vi "accuire.vi"() -> ()   [LabVIEW 2011]
uses:
  GUI_Template/GUI_master/tcp_new_data_event.ctl
  GUI_Template/GUI_master/tcp new data cluster.ctl
  Ctrs/beam detection.ctl
  GUI_Beampointing_single_TRA/Ctrs/move.ctl
  <userlib>/_OpenG.lib/array/array.llb/Filter 1D Array with Scalar (String)__ogtk.vi
  <vilib>/Analysis/NI_AALBase.lvlib
panel:
  in  "Offset X stats":dbl[][](array[numeric])
  in  "Offset Y stats":dbl[][](array[numeric])
  out "move properties 3":T1[](array[typedef])
  out "move properties 2":T1[](array[typedef])
  out "Box":T2(array[cluster])
  in  "Tab Control 2":enum32{"Config ", "Main", "History"}(tab)=enum."Main"
  in  "motor config":T3 {"Motor CCD 12" items=["PA2_Input1", "PA2_Input2", "L2_TelInpFar", "L1_TelInpNear", "L4_TREXPASS1", "L5_TREXPass2", "L6_TREXPass3", "L7_TREXPass4", "L8_M10Leak", "B1_TelInput", "B2_TelLens1", "", "", "", "MBeamSplitterL", "Mdiode"]; "Motor CCD 11" items=["PA2_Input1", "PA2_Input2", "L2_TelInpFar", "L1_TelInpNear", "L4_TREXPASS1", "L5_TREXPass2", "L6_TREXPass3", "L7_TREXPass4", "L8_M10Leak", "B1_TelInput", "B2_TelLens1", "", "", "", "MBeamSplitterL", "Mdiode"]; "Motor CCD 10" items=["PA2_Input1", "PA2_Input2", "L2_TelInpFar", "L1_TelInpNear", "L4_TREXPASS1", "L5_TREXPass2", "L6_TREXPass3", "L7_TREXPass4", "L8_M10Leak", "B1_TelInput", "B2_TelLens1", "", "", "", "MBeamSplitterL", "Mdiode"]; "Motor CCD 9" items=["PA2_Input1", "PA2_Input2", "L2_TelInpFar", "L1_TelInpNear", "L4_TREXPASS1", "L5_TREXPass2", "L6_TREXPass3", "L7_TREXPass4", "L8_M10Leak", "B1_TelInput", "B2_TelLens1", "", "", "", "MBeamSplitterL", "Mdiode"]; "Motor CCD 8" items=["PA2_Input1", "PA2_Input2", "L2_TelInpFar", "L1_TelInpNear", "L4_TREXPASS1", "L5_TREXPass2", "L6_TREXPass3", "L7_TREXPass4", "L8_M10Leak", "B1_TelInput", "B2_TelLens1", "", "", "", "MBeamSplitterL", "Mdiode"]; "Motor CCD 7" items=["PA2_Input1", "PA2_Input2", "L2_TelInpFar", "L1_TelInpNear", "L4_TREXPASS1", "L5_TREXPass2", "L6_TREXPass3", "L7_TREXPass4", "L8_M10Leak", "B1_TelInput", "B2_TelLens1", "", "", "", "MBeamSplitterL", "Mdiode"]; "Motor CCD 6" items=["PA2_Input1", "PA2_Input2", "L2_TelInpFar", "L1_TelInpNear", "L4_TREXPASS1", "L5_TREXPass2", "L6_TREXPass3", "L7_TREXPass4", "L8_M10Leak", "B1_TelInput", "B2_TelLens1", "", "", "", "MBeamSplitterL", "Mdiode"]; "Motor CCD 5" items=["PA2_Input1", "PA2_Input2", "L2_TelInpFar", "L1_TelInpNear", "L4_TREXPASS1", "L5_TREXPass2", "L6_TREXPass3", "L7_TREXPass4", "L8_M10Leak", "B1_TelInput", "B2_TelLens1", "", "", "", "MBeamSplitterL", "Mdiode"]; "Motor CCD 4" items=["PA2_Input1", "PA2_Input2", "L2_TelInpFar", "L1_TelInpNear", "L4_TREXPASS1", "L5_TREXPass2", "L6_TREXPass3", "L7_TREXPass4", "L8_M10Leak", "B1_TelInput", "B2_TelLens1", "", "", "", "MBeamSplitterL", "Mdiode"]; "Motor CCD 3" items=["PA2_Input1", "PA2_Input2", "L2_TelInpFar", "L1_TelInpNear", "L4_TREXPASS1", "L5_TREXPass2", "L6_TREXPass3", "L7_TREXPass4", "L8_M10Leak", "B1_TelInput", "B2_TelLens1", "", "", "", "MBeamSplitterL", "Mdiode"]; "Motor CCD 2" items=["PA2_Input1", "PA2_Input2", "L2_TelInpFar", "L1_TelInpNear", "L4_TREXPASS1", "L5_TREXPass2", "L6_TREXPass3", "L7_TREXPass4", "L8_M10Leak", "B1_TelInput", "B2_TelLens1", "", "", "", "MBeamSplitterL", "Mdiode"]; "Motor CCD 1" items=["PA2_Input1", "PA2_Input2", "L2_TelInpFar", "L1_TelInpNear", "L4_TREXPASS1", "L5_TREXPass2", "L6_TREXPass3", "L7_TREXPass4", "L8_M10Leak", "B1_TelInput", "B2_TelLens1", "", "", "", "MBeamSplitterL", "Mdiode"]}
  out "CCDs 2":T4
  out "sorted array X":cluster{dbl, "GUIdevice 7":string}[](array[cluster])
  out "sorted array Y":cluster{dbl, "GUIdevice 7":string}[](array[cluster])
  in  "Exposure::7":dbl=0.095 min=0.0001 max=1.0 format="%#_6f"
  in  "Triggerdelay::6":dbl=0.003 min=0.0 max=0.09 format="%#_6f"
  in  "Trigger::7":bool
  in  "Exposure::6":dbl=0.095 min=0.0001 max=1.0 format="%#_6f"
  in  "Triggerdelay::6":dbl=0.003 min=0.0 max=0.09 format="%#_6f"
  in  "Trigger::6":bool
  in  "Exposure::5":dbl=0.095 min=0.0001 max=1.0 format="%#_6f"
  in  "Triggerdelay::5":dbl=0.003 min=0.0 max=0.09 format="%#_6f"
  in  "Trigger::5":bool
  in  "Exposure::4":dbl=0.095 min=0.01 max=1.0 format="%#_6f"
  in  "Triggerdelay::4":dbl=0.003 min=0.0 max=0.09 format="%#_6f"
  in  "Trigger::4":bool
  in  "Exposure::3":dbl=0.095 min=0.0001 max=1.0 format="%#_6f"
  in  "Triggerdelay::3":dbl=0.003 min=0.0 max=0.09 format="%#_6f"
  in  "Trigger::3":bool
  in  "Exposure::2":dbl=0.095 min=0.0001 max=1.0 format="%#_6f"
  in  "Triggerdelay::2":dbl=0.003 min=0.0 max=0.09 format="%#_6f"
  in  "Trigger::2":bool
  out "image::1":T5(plugin-control) caption="L4_TREXpass1"
  out "image::2":T5(plugin-control) caption="L5_TREXPass2"
  out "image::3":T5(plugin-control) caption="L6_TREXpass3"
  out "image::4":T5(plugin-control) caption="L7_TREXPass4"
  out "image::5":T5(plugin-control) caption="L8_M10Leak"
  out "image::6":T5(plugin-control) caption="B1_TelInput"
  out "image::7":T5(plugin-control) caption="B2_TelLens1"
  out "Waveform Graph":cluster{i32, i32, "Centroid X":dbl[][]}(graph)
  out "image::8":T5(plugin-control)
  in  "Exposure::1":dbl=0.095 min=0.0001 max=1.0 format="%#_6f"
  in  "Triggerdelay::1":dbl=0.003 min=0.0 max=0.09 format="%#_6f"
  in  "Trigger::1":bool
  in  "UDP error message":string
  out "required Y":bool[](array[boolean])
  out "required X":bool[](array[boolean])
  out "detected":bool[](array[boolean])
  out "array":string[](array[string])
  out "CCD 5":cluster{timestamp[], dbl[]}[](graph)
  out "CCD 6":cluster{timestamp[], dbl[]}[](graph)
  out "CCD 7":cluster{timestamp[], dbl[]}[](graph)
  out "CCD 8":cluster{timestamp[], dbl[]}[](graph)
  out "CCD 1":cluster{timestamp[], dbl[]}[](graph)
  out "CCD 2":cluster{timestamp[], dbl[]}[](graph)
  out "CCD 3":cluster{timestamp[], dbl[]}[](graph)
  out "CCD 4":cluster{timestamp[], dbl[]}[](graph)
  in  "output cluster 2":T8 {"detection para"."smal para"."Measurement Parameter" items=["Center of Mass X", "Center of Mass Y", "First Pixel X", "First Pixel Y", "Bounding Rect Left", "Bounding Rect Top", "Bounding Rect Right", "Bounding Rect Bottom", "Max Feret Diameter Start X", "Max Feret Diameter Start Y", "Max Feret Diameter End X", "Max Feret Diameter End Y", "Max Horiz. Segment Length Left", "Max Horiz. Segment Length Right", "Max Horiz. Segment Length Row", "-", "Bounding Rect Width", "Bounding Rect Height", "Bounding Rect Diagonal", "Perimeter", "Convex Hull Perimeter", "Holes' Perimeter", "Max Feret Diameter", "Equivalent Ellipse Major Axis", "Equivalent Ellipse Minor Axis", "Equivalent Ellipse Minor Axis (Feret)", "Equivalent Rect Long Side", "Equivalent Rect Short Side", "Equivalent Rect Diagonal", "Equivalent Rect Short Side (Feret)", "Average Horiz. Segment Length", "Average Vert. Segment Length", "Hydraulic Radius", "Waddel Disk Diameter", "-", "Area", "Holes' Area", "Particle & Holes' Area", "Convex Hull Area", "Image Area", "-", "Number of Holes", "Number of Horiz. Segments", "Number of Vert. Segments", "-", "Orientation", "Max Feret Diameter Orientation", "-", "% Area/Image Area", "% Area/(Particle & Holes' Area)", "Ratio of Equivalent Ellipse Axes", "Ratio of Equivalent Rect Sides", "-", "Elongation Factor", "Compactness Factor", "Heywood Circularity Factor", "Type Factor", "-", "Sum X", "Sum Y", "Sum XX", "Sum XY", "Sum YY", "Sum XXX", "Sum XXY", "Sum XYY", "Sum YYY", "-", "Moment of Inertia XX", "Moment of Inertia XY", "Moment of Inertia YY", "Moment of Inertia XXX", "Moment of Inertia XXY", "Moment of Inertia XYY", "Moment of Inertia YYY", "Norm. Moment of Inertia XX", "Norm. Moment of Inertia XY", "Norm. Moment of Inertia YY", "Norm. Moment of Inertia XXX", "Norm. Moment of Inertia XXY", "Norm. Moment of Inertia XYY", "Norm. Moment of Inertia YYY", "Hu Moment 1", "Hu Moment 2", "Hu Moment 3", "Hu Moment 4", "Hu Moment 5", "Hu Moment 6", "Hu Moment 7"]; "detection para"."smal para"."Range Lower Value" format="%.2f"; "detection para"."smal para"."Range Upper Value" format="%.2f"; "detection para"."detection method" items=["clustering", "entropy", "metric", "moments", "inter-class variance"]; "detection para"."Filter" items=["No Filter", "Median Filter", "Low Pass Filter"]}
  out "Array":errorcluster[](array[cluster])
  out "Particle Reports (Pixels)":T9(array[cluster])
  in  "Feedback Global":bool
  in  "detection para":T6[](array[typedef])=[{"Filter"=1, "Filter Para"={"X Size"=5, "Y Size"=5, "% Tolerance"=1}, "detection method"=4, "smal para"=[{"Measurement Parameter"=35, "Range Lower Value"=0.0, "Range Upper Value"=0.0, "Range"=TRUE, "Measurement Type"=FALSE}], "Remove small Objects"=TRUE, "Restrict to round Objects"=FALSE}, {"Filter"=1, "Filter Para"={"X Size"=5, "Y Size"=5, "% Tolerance"=1}, "detection method"=4, "smal para"=[{"Measurement Parameter"=35, "Range Lower Value"=0.0, "Range Upper Value"=500.0, "Range"=FALSE, "Measurement Type"=FALSE}], "Remove small Objects"=TRUE, "Restrict to round Objects"=FALSE}, {"Filter"=1, "Filter Para"={"X Size"=5, "Y Size"=5, "% Tolerance"=1}, "detection method"=4, "smal para"=[{"Measurement Parameter"=35, "Range Lower Value"=0.0, "Range Upper Value"=500.0, "Range"=TRUE, "Measurement Type"=FALSE}], "Remove small Objects"=TRUE, "Restrict to round Objects"=FALSE}, {"Filter"=1, "Filter Para"={"X Size"=5, "Y Size"=5, "% Tolerance"=1}, "detection method"=4, "smal para"=[{"Measurement Parameter"=35, "Range Lower Value"=0.0, "Range Upper Value"=500.0, "Range"=TRUE, "Measurement Type"=FALSE}], "Remove small Objects"=TRUE, "Restrict to round Objects"=FALSE}, {"Filter"=1, "Filter Para"={"X Size"=5, "Y Size"=5, "% Tolerance"=1}, "detection method"=4, "smal para"=[{"Measurement Parameter"=35, "Range Lower Value"=0.0, "Range Upper Value"=500.0, "Range"=TRUE, "Measurement Type"=FALSE}], "Remove small Objects"=TRUE, "Restrict to round Objects"=FALSE}, {"Filter"=1, "Filter Para"={"X Size"=5, "Y Size"=5, "% Tolerance"=1}, "detection method"=4, "smal para"=[{"Measurement Parameter"=35, "Range Lower Value"=0.0, "Range Upper Value"=500.0, "Range"=TRUE, "Measurement Type"=FALSE}], "Remove small Objects"=TRUE, "Restrict to round Objects"=FALSE}, {"Filter"=1, "Filter Para"={"X Size"=5, "Y Size"=5, "% Tolerance"=1}, "detection method"=4, "smal para"=[{"Measurement Parameter"=35, "Range Lower Value"=0.0, "Range Upper Value"=500.0, "Range"=TRUE, "Measurement Type"=FALSE}], "Remove small Objects"=TRUE, "Restrict to round Objects"=FALSE}, {"Filter"=1, "Filter Para"={"X Size"=5, "Y Size"=5, "% Tolerance"=1}, "detection method"=3, "smal para"=[{"Measurement Parameter"=35, "Range Lower Value"=0.0, "Range Upper Value"=0.0, "Range"=FALSE, "Measurement Type"=FALSE}], "Remove small Objects"=TRUE, "Restrict to round Objects"=FALSE}, {"Filter"=1, "Filter Para"={"X Size"=5, "Y Size"=5, "% Tolerance"=1}, "detection method"=4, "smal para"=[{"Measurement Parameter"=35, "Range Lower Value"=0.0, "Range Upper Value"=0.0, "Range"=FALSE, "Measurement Type"=FALSE}], "Remove small Objects"=TRUE, "Restrict to round Objects"=FALSE}, {"Filter"=1, "Filter Para"={"X Size"=5, "Y Size"=5, "% Tolerance"=1}, "detection method"=4, "smal para"=[{"Measurement Parameter"=35, "Range Lower Value"=0.0, "Range Upper Value"=500.0, "Range"=TRUE, "Measurement Type"=FALSE}], "Remove small Objects"=TRUE, "Restrict to round Objects"=FALSE}, {"Filter"=1, "Filter Para"={"X Size"=5, "Y Size"=5, "% Tolerance"=1}, "detection method"=4, "smal para"=[{"Measurement Parameter"=35, "Range Lower Value"=0.0, "Range Upper Value"=500.0, "Range"=TRUE, "Measurement Type"=FALSE}], "Remove small Objects"=TRUE, "Restrict to round Objects"=FALSE}, {"Filter"=1, "Filter Para"={"X Size"=5, "Y Size"=5, "% Tolerance"=1}, "detection method"=4, "smal para"=[{"Measurement Parameter"=35, "Range Lower Value"=0.0, "Range Upper Value"=500.0, "Range"=TRUE, "Measurement Type"=FALSE}], "Remove small Objects"=TRUE, "Restrict to round Objects"=FALSE}] {"smal para"."Measurement Parameter" items=["Center of Mass X", "Center of Mass Y", "First Pixel X", "First Pixel Y", "Bounding Rect Left", "Bounding Rect Top", "Bounding Rect Right", "Bounding Rect Bottom", "Max Feret Diameter Start X", "Max Feret Diameter Start Y", "Max Feret Diameter End X", "Max Feret Diameter End Y", "Max Horiz. Segment Length Left", "Max Horiz. Segment Length Right", "Max Horiz. Segment Length Row", "-", "Bounding Rect Width", "Bounding Rect Height", "Bounding Rect Diagonal", "Perimeter", "Convex Hull Perimeter", "Holes' Perimeter", "Max Feret Diameter", "Equivalent Ellipse Major Axis", "Equivalent Ellipse Minor Axis", "Equivalent Ellipse Minor Axis (Feret)", "Equivalent Rect Long Side", "Equivalent Rect Short Side", "Equivalent Rect Diagonal", "Equivalent Rect Short Side (Feret)", "Average Horiz. Segment Length", "Average Vert. Segment Length", "Hydraulic Radius", "Waddel Disk Diameter", "-", "Area", "Holes' Area", "Particle & Holes' Area", "Convex Hull Area", "Image Area", "-", "Number of Holes", "Number of Horiz. Segments", "Number of Vert. Segments", "-", "Orientation", "Max Feret Diameter Orientation", "-", "% Area/Image Area", "% Area/(Particle & Holes' Area)", "Ratio of Equivalent Ellipse Axes", "Ratio of Equivalent Rect Sides", "-", "Elongation Factor", "Compactness Factor", "Heywood Circularity Factor", "Type Factor", "-", "Sum X", "Sum Y", "Sum XX", "Sum XY", "Sum YY", "Sum XXX", "Sum XXY", "Sum XYY", "Sum YYY", "-", "Moment of Inertia XX", "Moment of Inertia XY", "Moment of Inertia YY", "Moment of Inertia XXX", "Moment of Inertia XXY", "Moment of Inertia XYY", "Moment of Inertia YYY", "Norm. Moment of Inertia XX", "Norm. Moment of Inertia XY", "Norm. Moment of Inertia YY", "Norm. Moment of Inertia XXX", "Norm. Moment of Inertia XXY", "Norm. Moment of Inertia XYY", "Norm. Moment of Inertia YYY", "Hu Moment 1", "Hu Moment 2", "Hu Moment 3", "Hu Moment 4", "Hu Moment 5", "Hu Moment 6", "Hu Moment 7"]; "smal para"."Range Lower Value" format="%.2f"; "smal para"."Range Upper Value" format="%.2f"; "detection method" items=["clustering", "entropy", "metric", "moments", "inter-class variance"]; "Filter" items=["No Filter", "Median Filter", "Low Pass Filter"]}
  in  "Target.X::8":dbl=47.0 min=0.0 max=2000.0 format="%#_6f"
  in  "Target.Y::8":dbl=45.0 min=0.0 max=2000.0 format="%#_6f"
  in  "GUIdevice 8":string
  in  "Tab Control":T10(tab)=enum."Detection"
  in  "Save Stats":bool
  in  "Save Config":bool
  in  "Load Config":bool
  in  "updat speed [ms]":i32=200
  in  "img to avg":i32=20
  in  "Reset History":bool
  in  "beam detection para":T6={"Filter"=1, "Filter Para"={"X Size"=5, "Y Size"=5, "% Tolerance"=1}, "detection method"=4, "smal para"=[{"Measurement Parameter"=35, "Range Lower Value"=0.0, "Range Upper Value"=500.0, "Range"=FALSE, "Measurement Type"=FALSE}], "Remove small Objects"=TRUE, "Restrict to round Objects"=FALSE} {"smal para"."Measurement Parameter" items=["Center of Mass X", "Center of Mass Y", "First Pixel X", "First Pixel Y", "Bounding Rect Left", "Bounding Rect Top", "Bounding Rect Right", "Bounding Rect Bottom", "Max Feret Diameter Start X", "Max Feret Diameter Start Y", "Max Feret Diameter End X", "Max Feret Diameter End Y", "Max Horiz. Segment Length Left", "Max Horiz. Segment Length Right", "Max Horiz. Segment Length Row", "-", "Bounding Rect Width", "Bounding Rect Height", "Bounding Rect Diagonal", "Perimeter", "Convex Hull Perimeter", "Holes' Perimeter", "Max Feret Diameter", "Equivalent Ellipse Major Axis", "Equivalent Ellipse Minor Axis", "Equivalent Ellipse Minor Axis (Feret)", "Equivalent Rect Long Side", "Equivalent Rect Short Side", "Equivalent Rect Diagonal", "Equivalent Rect Short Side (Feret)", "Average Horiz. Segment Length", "Average Vert. Segment Length", "Hydraulic Radius", "Waddel Disk Diameter", "-", "Area", "Holes' Area", "Particle & Holes' Area", "Convex Hull Area", "Image Area", "-", "Number of Holes", "Number of Horiz. Segments", "Number of Vert. Segments", "-", "Orientation", "Max Feret Diameter Orientation", "-", "% Area/Image Area", "% Area/(Particle & Holes' Area)", "Ratio of Equivalent Ellipse Axes", "Ratio of Equivalent Rect Sides", "-", "Elongation Factor", "Compactness Factor", "Heywood Circularity Factor", "Type Factor", "-", "Sum X", "Sum Y", "Sum XX", "Sum XY", "Sum YY", "Sum XXX", "Sum XXY", "Sum XYY", "Sum YYY", "-", "Moment of Inertia XX", "Moment of Inertia XY", "Moment of Inertia YY", "Moment of Inertia XXX", "Moment of Inertia XXY", "Moment of Inertia XYY", "Moment of Inertia YYY", "Norm. Moment of Inertia XX", "Norm. Moment of Inertia XY", "Norm. Moment of Inertia YY", "Norm. Moment of Inertia XXX", "Norm. Moment of Inertia XXY", "Norm. Moment of Inertia XYY", "Norm. Moment of Inertia YYY", "Hu Moment 1", "Hu Moment 2", "Hu Moment 3", "Hu Moment 4", "Hu Moment 5", "Hu Moment 6", "Hu Moment 7"]; "smal para"."Range Lower Value" format="%.2f"; "smal para"."Range Upper Value" format="%.2f"; "detection method" items=["clustering", "entropy", "metric", "moments", "inter-class variance"]; "Filter" items=["No Filter", "Median Filter", "Low Pass Filter"]}
  in  "move config":T1={"Tolerance [%]"=0.1, "Stepsize"=0.0001, "Invert Axis"=TRUE, "Invert Direction X"=FALSE, "Invert Direction Y"=TRUE, "enable feedback"=FALSE, "my activ motor"=""}
  out "Arguments Y":string
  in  "active axis refs 2":T11(array[cluster])
  in  "active Axis ref":cluster{"Ref X":refnum<vi>, "Ref Y":refnum<vi>}
  in  "CCDs":u16(ring) items=["L4_TREXpass1", "L5_TREXPass2", "L6_TREXpass3", "L7_TREXPass4", "L8_M10Leak", "B1_TelInput", "B2_TelLens1", ""]
  out "motor refs":refnum<vi>[](array[refnum])
  in  "Position.Axis 511::99":dbl=77.0 caption="Motor Axis 1" min=-999999.0 max=999999.0 format="%#_6f"
  in  "Position.Axis 512::99":dbl=77.0 caption="Motor Axis 1" min=-999999.0 max=999999.0 format="%#_6f"
  in  "Position.Axis 513::99":dbl=77.0 caption="Motor Axis 1" min=-999999.0 max=999999.0 format="%#_6f"
  in  "Position.Axis 521::99":dbl=77.0 caption="Motor Axis 1" min=-999999.0 max=999999.0 format="%#_6f"
  in  "Position.Axis 522::99":dbl=77.0 caption="Motor Axis 1" min=-999999.0 max=999999.0 format="%#_6f"
  in  "Position.Axis 523::99":dbl=77.0 caption="Motor Axis 1" min=-999999.0 max=999999.0 format="%#_6f"
  in  "Position.Axis 531::99":dbl=77.0 caption="Motor Axis 1" min=-999999.0 max=999999.0 format="%#_6f"
  in  "Position.Axis 532::99":dbl=77.0 caption="Motor Axis 1" min=-999999.0 max=999999.0 format="%#_6f"
  in  "Position.Axis 533::99":dbl=77.0 caption="Motor Axis 1" min=-999999.0 max=999999.0 format="%#_6f"
  in  "Position.Axis 541::99":dbl=77.0 caption="Motor Axis 1" min=-999999.0 max=999999.0 format="%#_6f"
  in  "Position.Axis 542::99":dbl=77.0 caption="Motor Axis 1" min=-999999.0 max=999999.0 format="%#_6f"
  in  "Position.Axis 543::99":dbl=77.0 caption="Motor Axis 1" min=-999999.0 max=999999.0 format="%#_6f"
  in  "Position.Axis 411::99":dbl=77.0 caption="Motor Axis 1" min=-999999.0 max=999999.0 format="%#_6f"
  in  "Position.Axis 412::99":dbl=77.0 caption="Motor Axis 1" min=-999999.0 max=999999.0 format="%#_6f"
  in  "Position.Axis 413::99":dbl=77.0 caption="Motor Axis 1" min=-999999.0 max=999999.0 format="%#_6f"
  in  "Position.Axis 421::99":dbl=77.0 caption="Motor Axis 1" min=-999999.0 max=999999.0 format="%#_6f"
  in  "Position.Axis 422::99":dbl=77.0 caption="Motor Axis 1" min=-999999.0 max=999999.0 format="%#_6f"
  in  "Position.Axis 423::99":dbl=77.0 caption="Motor Axis 1" min=-999999.0 max=999999.0 format="%#_6f"
  in  "Position.Axis 431::99":dbl=77.0 caption="Motor Axis 1" min=-999999.0 max=999999.0 format="%#_6f"
  in  "Position.Axis 432::99":dbl=77.0 caption="Motor Axis 1" min=-999999.0 max=999999.0 format="%#_6f"
  in  "Position.Axis 433::99":dbl=77.0 caption="Motor Axis 1" min=-999999.0 max=999999.0 format="%#_6f"
  in  "Position.Axis 441::99":dbl=77.0 caption="Motor Axis 1" min=-999999.0 max=999999.0 format="%#_6f"
  in  "Position.Axis 442::99":dbl=77.0 caption="Motor Axis 1" min=-999999.0 max=999999.0 format="%#_6f"
  in  "Position.Axis 443::99":dbl=77.0 caption="Motor Axis 1" min=-999999.0 max=999999.0 format="%#_6f"
  in  "Position.Axis 311::99":dbl=77.0 caption="Motor Axis 1" min=-999999.0 max=999999.0 format="%#_6f"
  in  "Position.Axis 312::99":dbl=77.0 caption="Motor Axis 1" min=-999999.0 max=999999.0 format="%#_6f"
  in  "Position.Axis 313::99":dbl=77.0 caption="Motor Axis 1" min=-999999.0 max=999999.0 format="%#_6f"
  in  "Position.Axis 321::99":dbl=77.0 caption="Motor Axis 1" min=-999999.0 max=999999.0 format="%#_6f"
  in  "Position.Axis 322::99":dbl=77.0 caption="Motor Axis 1" min=-999999.0 max=999999.0 format="%#_6f"
  in  "Position.Axis 323::99":dbl=77.0 caption="Motor Axis 1" min=-999999.0 max=999999.0 format="%#_6f"
  in  "Position.Axis 331::99":dbl=77.0 caption="Motor Axis 1" min=-999999.0 max=999999.0 format="%#_6f"
  in  "Position.Axis 332::99":dbl=77.0 caption="Motor Axis 1" min=-999999.0 max=999999.0 format="%#_6f"
  in  "Position.Axis 333::99":dbl=77.0 caption="Motor Axis 1" min=-999999.0 max=999999.0 format="%#_6f"
  in  "Position.Axis 341::99":dbl=77.0 caption="Motor Axis 1" min=-999999.0 max=999999.0 format="%#_6f"
  in  "Position.Axis 342::99":dbl=77.0 caption="Motor Axis 1" min=-999999.0 max=999999.0 format="%#_6f"
  in  "Position.Axis 343::99":dbl=77.0 caption="Motor Axis 1" min=-999999.0 max=999999.0 format="%#_6f"
  in  "Position.Axis 241::99":dbl=77.0 caption="Motor Axis 1" min=-999999.0 max=999999.0 format="%#_6f"
  in  "Position.Axis 242::99":dbl=77.0 caption="Motor Axis 1" min=-999999.0 max=999999.0 format="%#_6f"
  in  "Position.Axis 243::99":dbl=77.0 caption="Motor Axis 1" min=-999999.0 max=999999.0 format="%#_6f"
  in  "Position.Axis 231::99":dbl=77.0 caption="Motor Axis 1" min=-999999.0 max=999999.0 format="%#_6f"
  in  "Position.Axis 232::99":dbl=77.0 caption="Motor Axis 1" min=-999999.0 max=999999.0 format="%#_6f"
  in  "Position.Axis 233::99":dbl=77.0 caption="Motor Axis 1" min=-999999.0 max=999999.0 format="%#_6f"
  in  "Position.Axis 221::99":dbl=77.0 caption="Motor Axis 1" min=-20000.0 max=20000.0 format="%#_6f"
  in  "Position.Axis 222::99":dbl=77.0 caption="Motor Axis 1" min=-200000.0 max=200000.0 format="%#_6f"
  in  "Position.Axis 223::99":dbl=77.0 caption="Motor Axis 1" min=-20000.0 max=200000000.0 format="%#_6f"
  in  "Position.Axis 211::99":dbl=77.0 caption="Motor Axis 1" min=-200000.0 max=2000000.0 format="%#_6f"
  in  "Position.Axis 212::99":dbl=77.0 caption="Motor Axis 1" min=-200000.0 max=2000.0 format="%#_6f"
  in  "Position.Axis 213::99":dbl=77.0 caption="Motor Axis 1" min=-2000.0 max=2000000.0 format="%#_6f"
  in  "Position.Axis 141::99":dbl=77.0 caption="Motor Axis 1" min=-999999.0 max=999999.0 format="%#_6f"
  in  "Position.Axis 142::99":dbl=77.0 caption="Motor Axis 1" min=-999999.0 max=999999.0 format="%#_6f"
  in  "Position.Axis 143::99":dbl=77.0 caption="Motor Axis 1" min=-999999.0 max=999999.0 format="%#_6f"
  in  "Position.Axis 131::99":dbl=77.0 caption="Motor Axis 1" min=-999999.0 max=999999.0 format="%#_6f"
  in  "Position.Axis 132::99":dbl=77.0 caption="Motor Axis 1" min=-999999.0 max=999999.0 format="%#_6f"
  in  "Position.Axis 133::99":dbl=77.0 caption="Motor Axis 1" min=-999999.0 max=999999.0 format="%#_6f"
  in  "Position.Axis 121::99":dbl=77.0 caption="Motor Axis 1" min=-999999.0 max=999999.0 format="%#_6f"
  in  "Position.Axis 122::99":dbl=77.0 caption="Motor Axis 1" min=-999999.0 max=999999.0 format="%#_6f"
  in  "Position.Axis 123::99":dbl=77.0 caption="Motor Axis 1" min=-999999.0 max=999999.0 format="%#_6f"
  in  "Position.Axis 113::99":dbl=77.0 caption="Motor Axis 1" min=-999999.0 max=999999.0 format="%#_6f"
  in  "Position.Axis 112::99":dbl=77.0 caption="Motor Axis 1" min=-999999.0 max=999999.0 format="%#_6f"
  in  "Position.Axis 111::99":dbl=77.0 caption="Motor Axis 1" min=-999999.0 max=999999.0 format="%#_6f"
  out "Arguments X":string
  in  "GUIdevice 99":string="PicoPad3"
  in  "move properties":T1[](array[typedef])=[{"Tolerance [%]"=5.0, "Stepsize"=5.0, "Invert Axis"=FALSE, "Invert Direction X"=FALSE, "Invert Direction Y"=FALSE, "enable feedback"=FALSE, "my activ motor"=""}, {"Tolerance [%]"=5.0, "Stepsize"=5.0, "Invert Axis"=FALSE, "Invert Direction X"=FALSE, "Invert Direction Y"=FALSE, "enable feedback"=FALSE, "my activ motor"=""}, {"Tolerance [%]"=5.0, "Stepsize"=5.0, "Invert Axis"=FALSE, "Invert Direction X"=FALSE, "Invert Direction Y"=FALSE, "enable feedback"=FALSE, "my activ motor"=""}, {"Tolerance [%]"=5.0, "Stepsize"=5.0, "Invert Axis"=FALSE, "Invert Direction X"=FALSE, "Invert Direction Y"=FALSE, "enable feedback"=FALSE, "my activ motor"=""}, {"Tolerance [%]"=5.0, "Stepsize"=5.0, "Invert Axis"=FALSE, "Invert Direction X"=FALSE, "Invert Direction Y"=FALSE, "enable feedback"=FALSE, "my activ motor"=""}, {"Tolerance [%]"=5.0, "Stepsize"=5.0, "Invert Axis"=FALSE, "Invert Direction X"=FALSE, "Invert Direction Y"=FALSE, "enable feedback"=FALSE, "my activ motor"=""}, {"Tolerance [%]"=5.0, "Stepsize"=5.0, "Invert Axis"=FALSE, "Invert Direction X"=FALSE, "Invert Direction Y"=FALSE, "enable feedback"=FALSE, "my activ motor"=""}, {"Tolerance [%]"=5.0, "Stepsize"=5.0, "Invert Axis"=FALSE, "Invert Direction X"=FALSE, "Invert Direction Y"=FALSE, "enable feedback"=FALSE, "my activ motor"=""}, {"Tolerance [%]"=5.0, "Stepsize"=5.0, "Invert Axis"=FALSE, "Invert Direction X"=FALSE, "Invert Direction Y"=FALSE, "enable feedback"=FALSE, "my activ motor"=""}, {"Tolerance [%]"=5.0, "Stepsize"=5.0, "Invert Axis"=FALSE, "Invert Direction X"=FALSE, "Invert Direction Y"=FALSE, "enable feedback"=FALSE, "my activ motor"=""}, {"Tolerance [%]"=5.0, "Stepsize"=5.0, "Invert Axis"=FALSE, "Invert Direction X"=FALSE, "Invert Direction Y"=FALSE, "enable feedback"=FALSE, "my activ motor"=""}, {"Tolerance [%]"=5.0, "Stepsize"=5.0, "Invert Axis"=FALSE, "Invert Direction X"=FALSE, "Invert Direction Y"=FALSE, "enable feedback"=FALSE, "my activ motor"=""}, {"Tolerance [%]"=5.0, "Stepsize"=5.0, "Invert Axis"=FALSE, "Invert Direction X"=FALSE, "Invert Direction Y"=FALSE, "enable feedback"=FALSE, "my activ motor"=""}]
  in  "Time":timestamp[][](array[timestamp])
  in  "Mean Size":dbl[][](array[numeric])
  in  "Size":dbl[][](array[numeric])
  in  "active CCDs":i32(listbox)=1
  in  "Offset Y":dbl[][](array[numeric])
  in  "Offset X":dbl[][](array[numeric])
  in  "Mean Centroid X":dbl[][](array[numeric])
  in  "Mean Centroid Y":dbl[][](array[numeric])
  in  "Centroid Y":dbl[][](array[numeric])
  in  "Centroid X":dbl[][](array[numeric])
  in  "Target.X::7":dbl=47.0 min=0.0 max=2000.0 format="%#_6f"
  in  "Target.Y::7":dbl=45.0 min=0.0 max=2000.0 format="%#_6f"
  in  "Target.X::6":dbl=47.0 min=0.0 max=2000.0 format="%#_6f"
  in  "Target.Y::6":dbl=45.0 min=0.0 max=2000.0 format="%#_6f"
  in  "Target.X::5":dbl=47.0 min=0.0 max=2000.0 format="%#_6f"
  in  "Target.Y::5":dbl=45.0 min=0.0 max=2000.0 format="%#_6f"
  in  "Target.X::4":dbl=47.0 min=0.0 max=2000.0 format="%#_6f"
  in  "Target.Y::4":dbl=45.0 min=0.0 max=2000.0 format="%#_6f"
  in  "Target.X::3":dbl=152.0 min=0.0 max=2000.0 format="%#_6f"
  in  "Target.Y::3":dbl=163.0 min=0.0 max=2000.0 format="%#_6f"
  in  "Target.X::2":dbl=75.0 min=0.0 max=2000.0 format="%#_6f"
  in  "Target.Y::2":dbl=74.0 min=0.0 max=2000.0 format="%#_6f"
  in  "Target.X::1":dbl=77.0 min=0.0 max=2000.0 format="%#_6f"
  in  "Target.Y::1":dbl=61.0 min=0.0 max=2000.0 format="%#_6f"
  in  "GUIdevice 7":string="B2_TelLens1"
  in  "GUIdevice 6":string="B1_TelInput"
  in  "GUIdevice 5":string="L8_M10Leak"
  in  "GUIdevice 4":string="L7_TREXPass4"
  in  "GUIdevice 3":string="L6_TREXpass3"
  in  "GUIdevice 2":string="L5_TREXPass2"
  in  "insert tag":bool=TRUE
  in  "stop":bool
  in  "GUIdevice 1":string="L4_TREXpass1"
  out "tcp data event":T12
  out "error IO 2":errorcluster
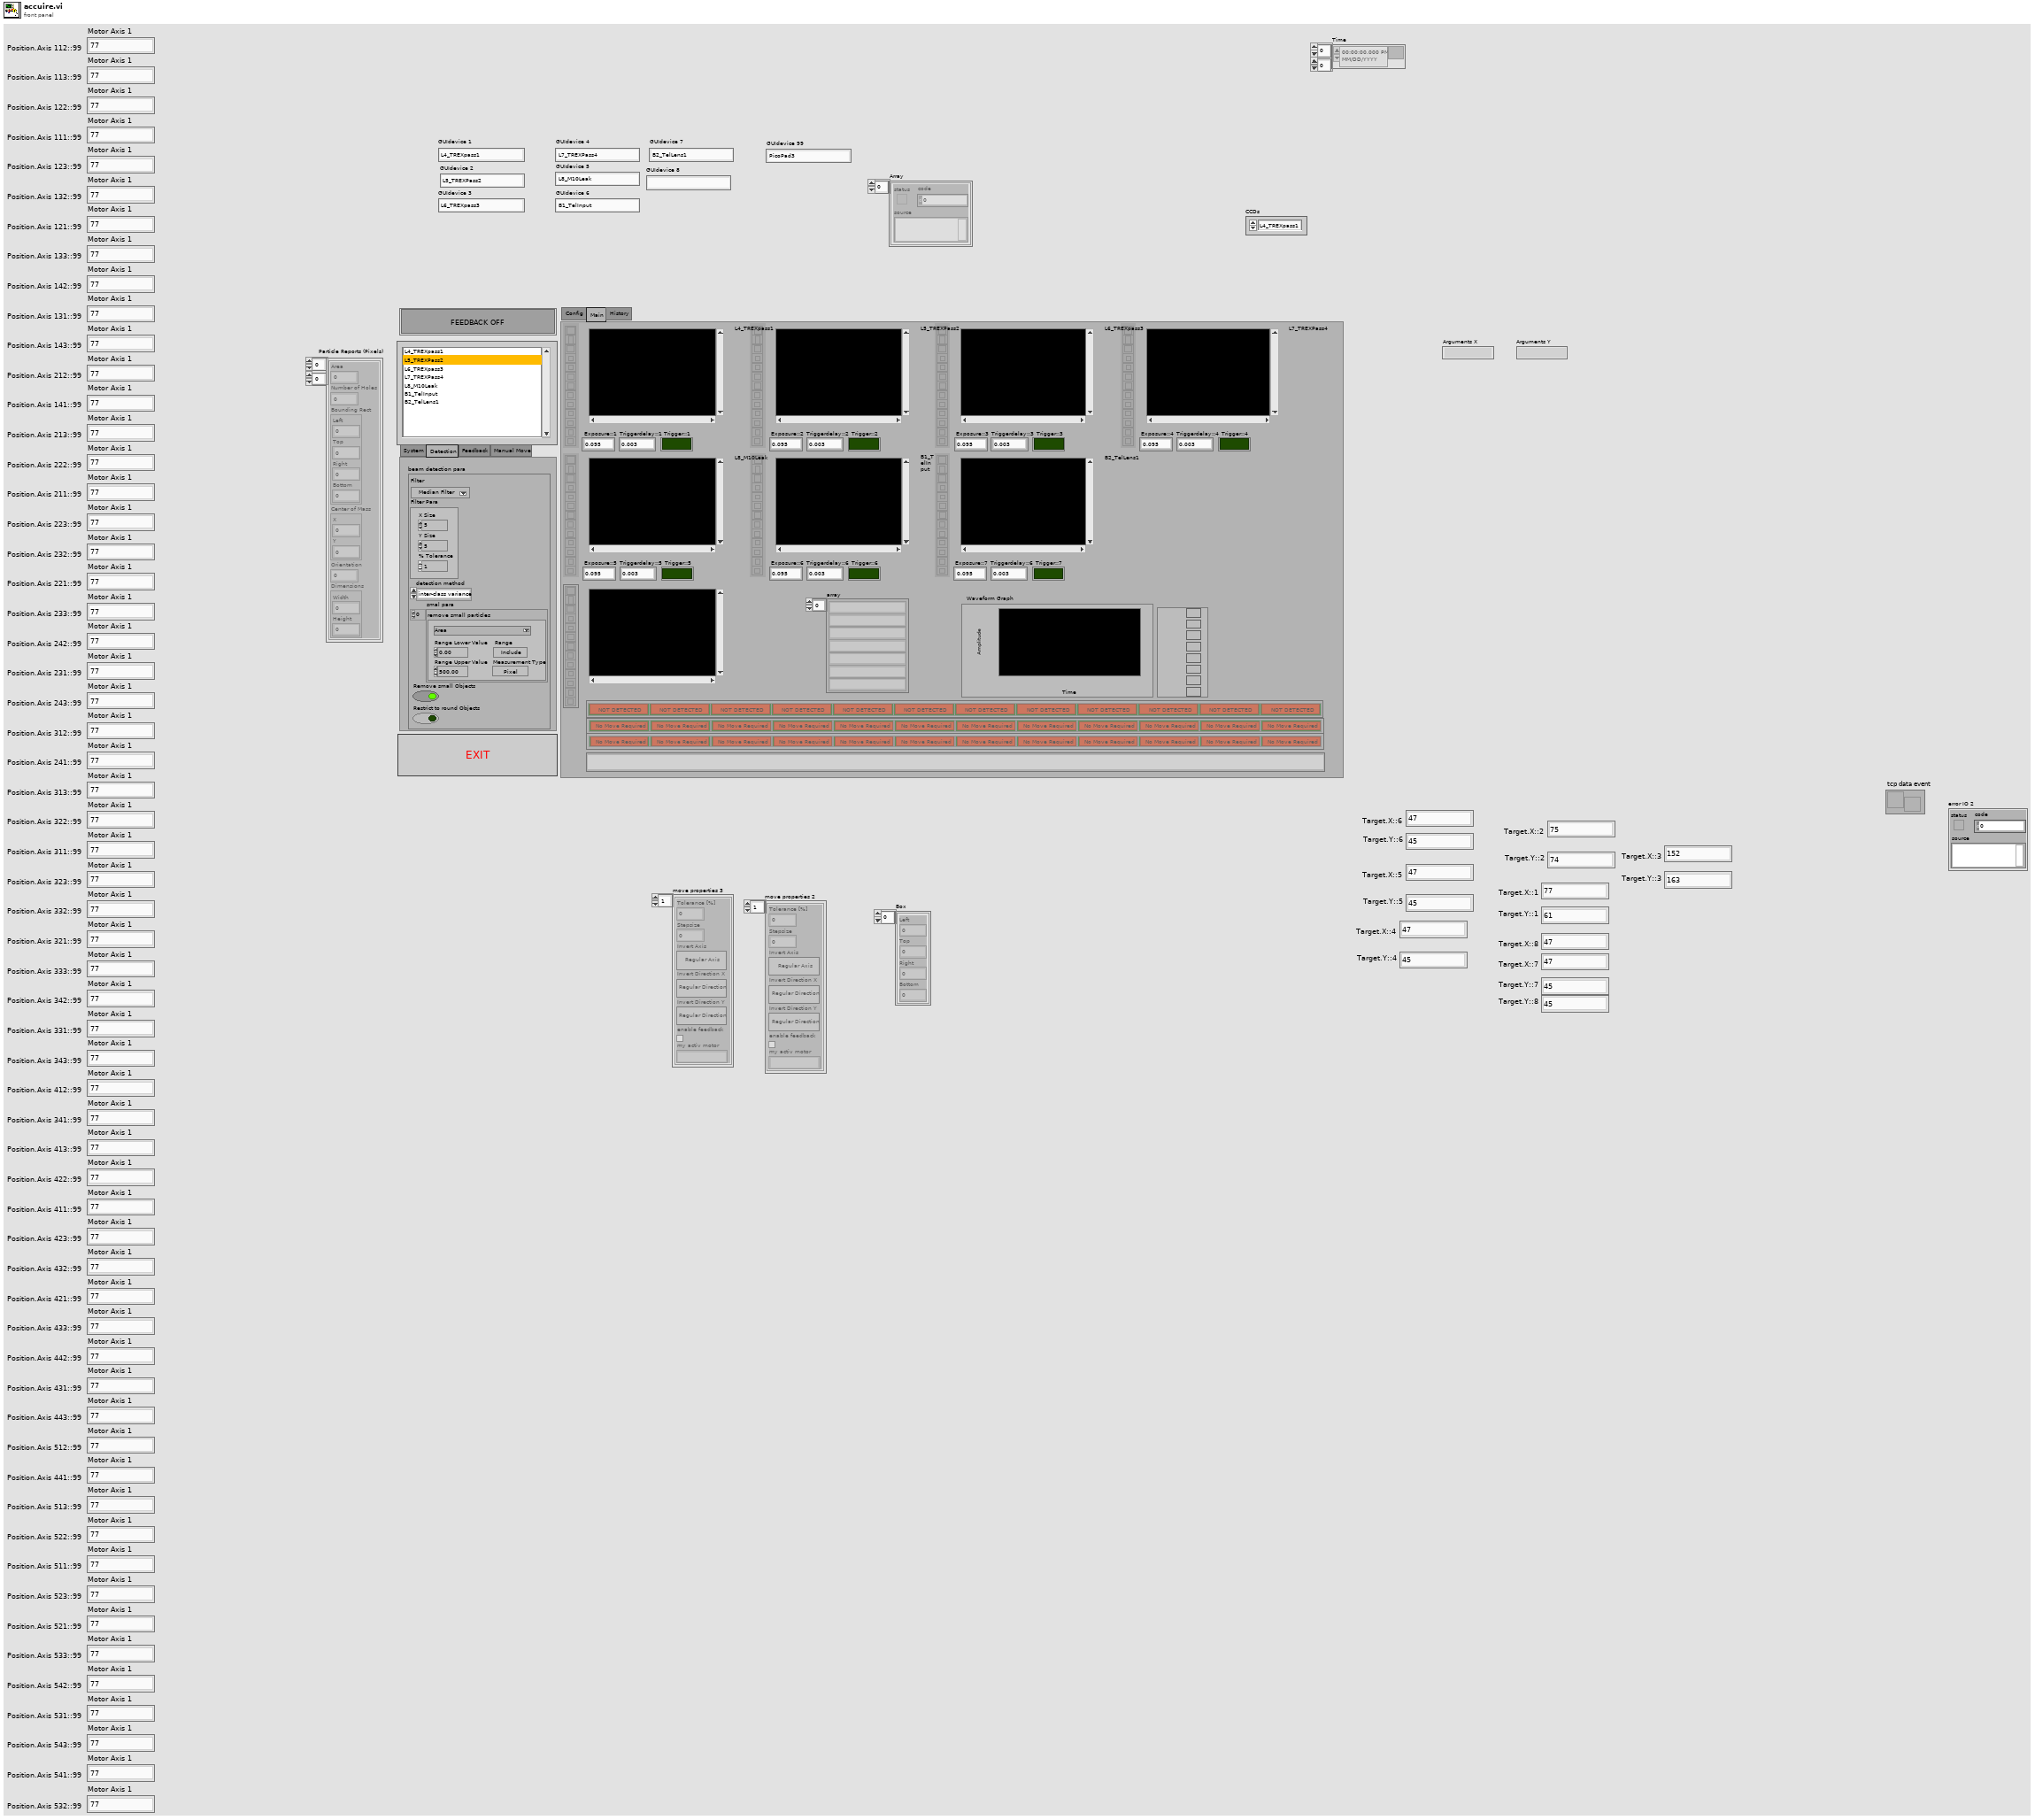
[diagram p1: front panel]
types:
  T1 = typedef "move.ctl" = cluster{"Tolerance [%]":dbl, "Stepsize":dbl, "Invert Axis":bool, "Invert Direction X":bool, "Invert Direction Y":bool, "enable feedback":bool, "my activ motor":string}
  T2 = cluster{"Left":dbl, "Top":dbl, "Right":dbl, "Bottom":dbl}[]
  T3 = cluster{"Motor CCD 1":u16, "Motor CCD 2":u16, "Motor CCD 3":u16, "Motor CCD 4":u16, "Motor CCD 5":u16, "Motor CCD 6":u16, "Motor CCD 7":u16, "Motor CCD 8":u16, "Motor CCD 9":u16, "Motor CCD 10":u16, "Motor CCD 11":u16, "Motor CCD 12":u16}
  T4 = cluster{"[0]":string, "[1]":string, "[2]":string, "[3]":string, "[4]":string, "[5]":string, "[6]":string, "[7]":string, "[8]":string}
  T5 = typedef "IMAQ Image.ctl" = refnum<image>
  T6 = typedef "beam detection.ctl" = cluster{"Filter":u16, "Filter Para":cluster{"X Size":i32, "Y Size":i32, "% Tolerance":i32}, "detection method":i32, "smal para":cluster{"Measurement Parameter":T7, "Range Lower Value":dbl, "Range Upper Value":dbl, "Range":bool, "Measurement Type":bool}[], "Remove small Objects":bool, "Restrict to round Objects":bool}
  T7 = typedef "Particle Parameters" = i32
  T8 = cluster{"move properties":T1[], "detection para":T6[], "Value":cluster{"Motor CCD 1":u16, "Motor CCD 2":u16, "Motor CCD 3":u16, "Motor CCD 4":u16, "Motor CCD 5":u16, "Motor CCD 6":u16, "Motor CCD 7":u16, "Motor CCD 8":u16, "Motor CCD 9":u16, "Motor CCD 10":u16, "Motor CCD 11":u16, "Motor CCD 12":u16}}
  T9 = cluster{"Area":dbl, "Number of Holes":dbl, "Bounding Rect":cluster{"Left":dbl, "Top":dbl, "Right":dbl, "Bottom":dbl}, "Center of Mass":cluster{"X":dbl, "Y":dbl}, "Orientation":dbl, "Dimensions":cluster{"Width":dbl, "Height":dbl}}[][]
  T10 = enum32{"System", "Detection", "Feedback", "Manual Move"}
  T11 = cluster{"Ref X":refnum<vi>, "Ref Y":refnum<vi>}[]
  T12 = typedef "tcp_new_data_event.ctl" = refnum<user-event>
  T13 = typedef "Image Type" = u32
  T14 = typedef "tcp new data cluster.ctl" = cluster{"EventEnum":enum16{"new data", "connection status update"}, "Device name":string}
  T15 = cluster{"Target.X::1":refnum<vi>, "Target.Y::1":refnum<vi>}
  T16 = cluster{"Target.X::2":refnum<vi>, "Target.Y::2":refnum<vi>}
  T17 = cluster{"Target.X::3":refnum<vi>, "Target.Y::3":refnum<vi>}
  T18 = cluster{"Target.X::4":refnum<vi>, "Target.Y::4":refnum<vi>}
  T19 = cluster{"Target.X::5":refnum<vi>, "Target.Y::5":refnum<vi>}
  T20 = cluster{"Target.X::6":refnum<vi>, "Target.Y::6":refnum<vi>}
  T21 = cluster{"Target.X::7":refnum<vi>, "Target.Y::7":refnum<vi>}
  T22 = cluster{"Target.X::8":refnum<vi>, "Target.Y::8":refnum<vi>}
  T23 = cluster{"Target.X::8":refnum<vi>, "Target.Y::8":refnum<vi>}[]
  T24 = cluster{"Left":i32, "Top":i32, "Right":i32, "Bottom":i32}
  T25 = enum32{"invalid app kind", "Development System", "Run Time System", "Student Edition", "Embedded LabVIEW", "Evaluation", "Custom"}
  T26 = enum32{"Invalid", "Standard", "Closed", "Hidden", "Minimized", "Maximized"}
  T27 = enum16{"open", "replace", "create", "open or create", "replace or create", "replace or create with confirmation"}
  T28 = cluster{"Left":dbl, "Top":dbl, "Right":dbl, "Bottom":dbl}
  T29 = cluster{"Area":dbl, "Number of Holes":dbl, "Bounding Rect":cluster{"Left":dbl, "Top":dbl, "Right":dbl, "Bottom":dbl}, "Center of Mass":cluster{"X":dbl, "Y":dbl}, "Orientation":dbl, "Dimensions":cluster{"Width":dbl, "Height":dbl}}[]
  T30 = cluster{"Core":cluster{"Current VI Reference":refnum<vi>, "Close Panel on Exit?":bool}, "detection para":T6[], "Centroid X":dbl[][], "Centroid Y":dbl[][], "img to avg":i32, "Mean Centroid X":dbl[][], "Mean Centroid Y":dbl[][], "Offset X":dbl[][], "Offset Y":dbl[][], "Offset X stats ":dbl[][], "Offset Y stats ":dbl[][], "Size":dbl[][], "Mean Size":dbl[][], "Time":timestamp[][], "move properties":T1[], "active axis refs 2":cluster{"Ref X":refnum<vi>, "Ref Y":refnum<vi>}[], "active ccd":i32, "Feedback global":bool}
  T31 = cluster{"Current VI Reference":refnum<vi>, "Close Panel on Exit?":bool}
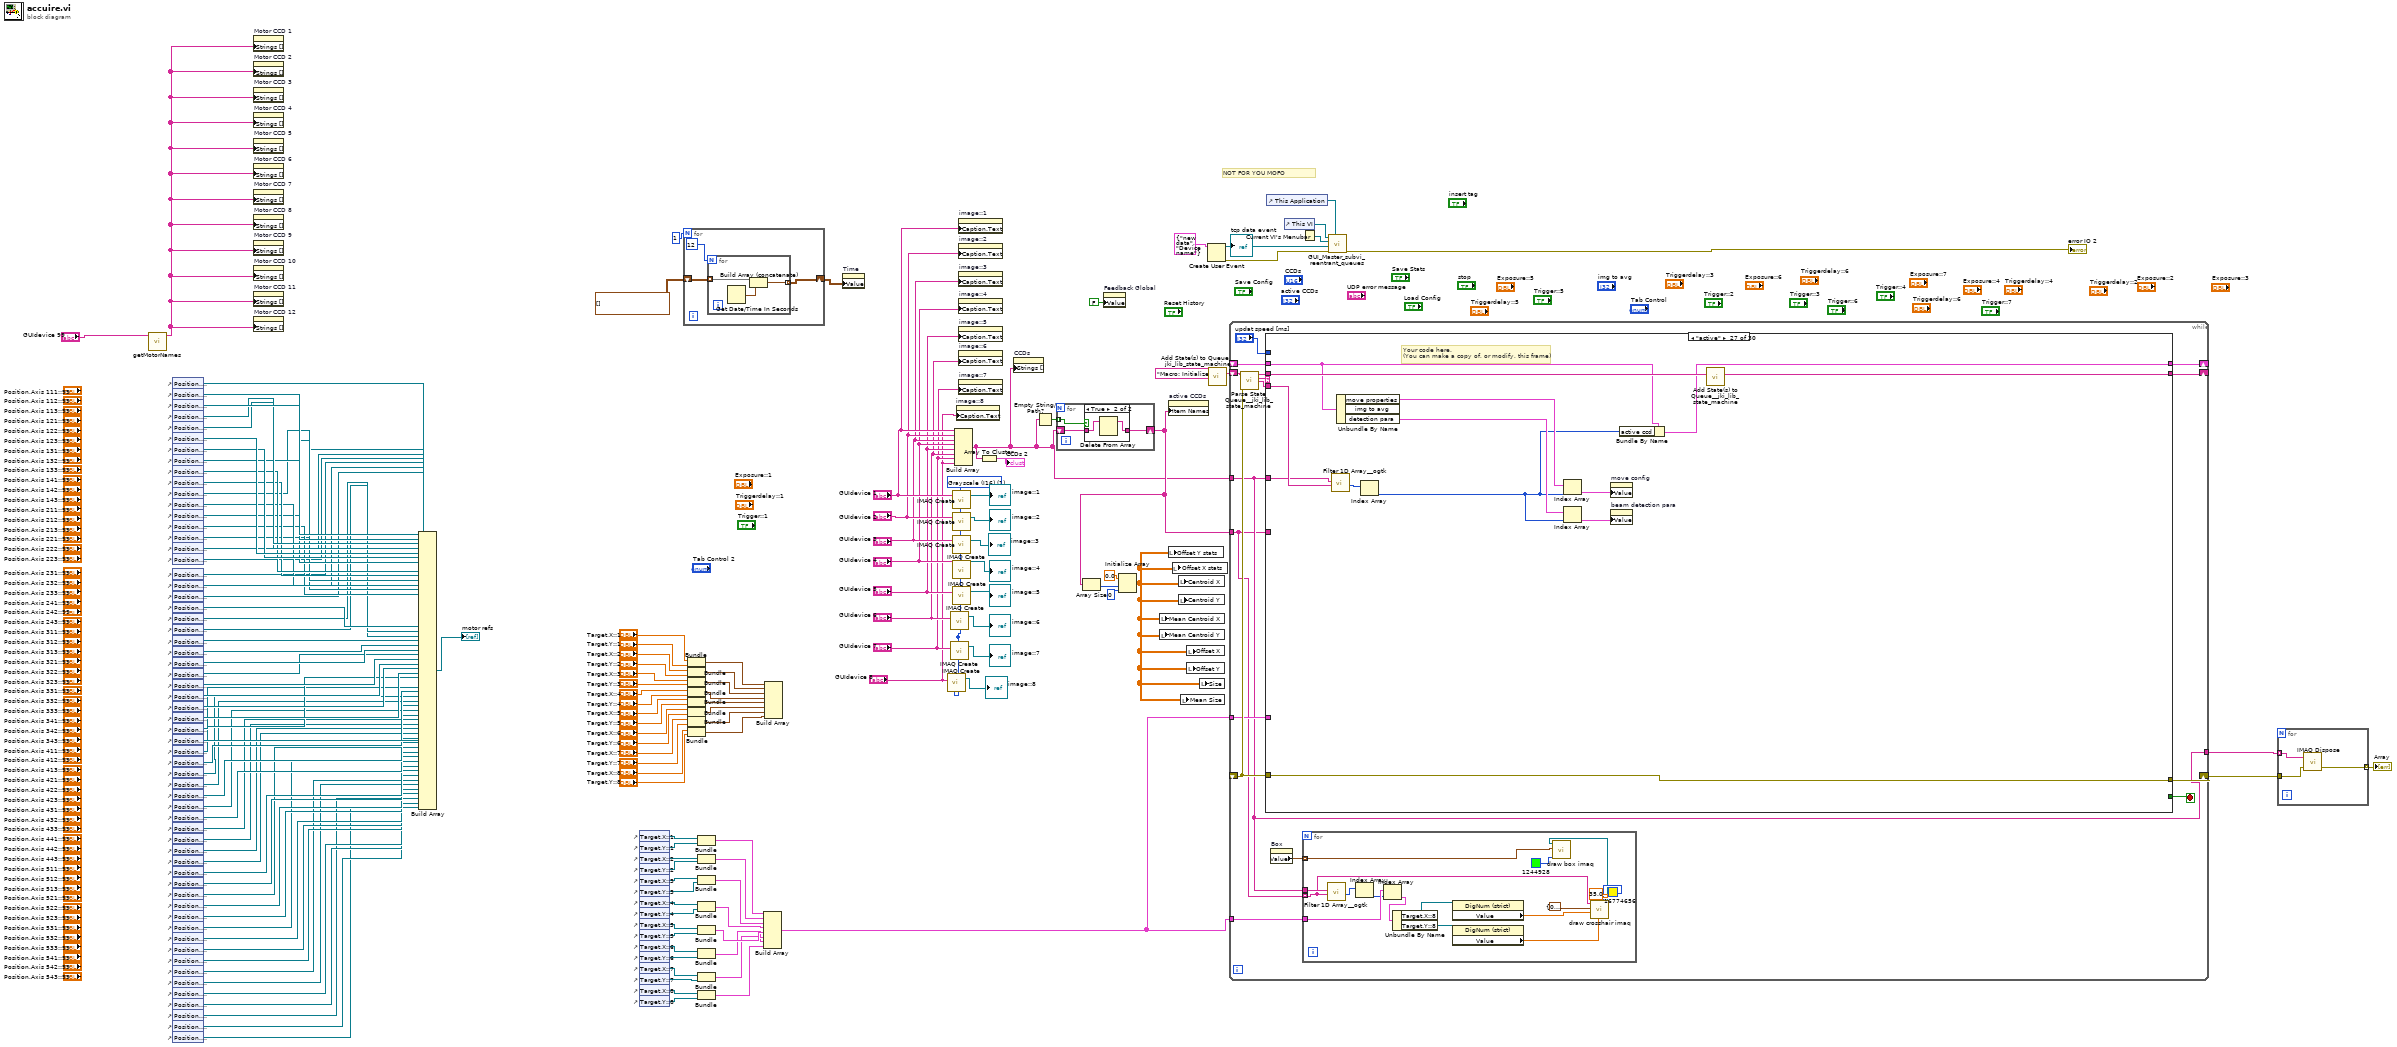
[diagram p0: block diagram]
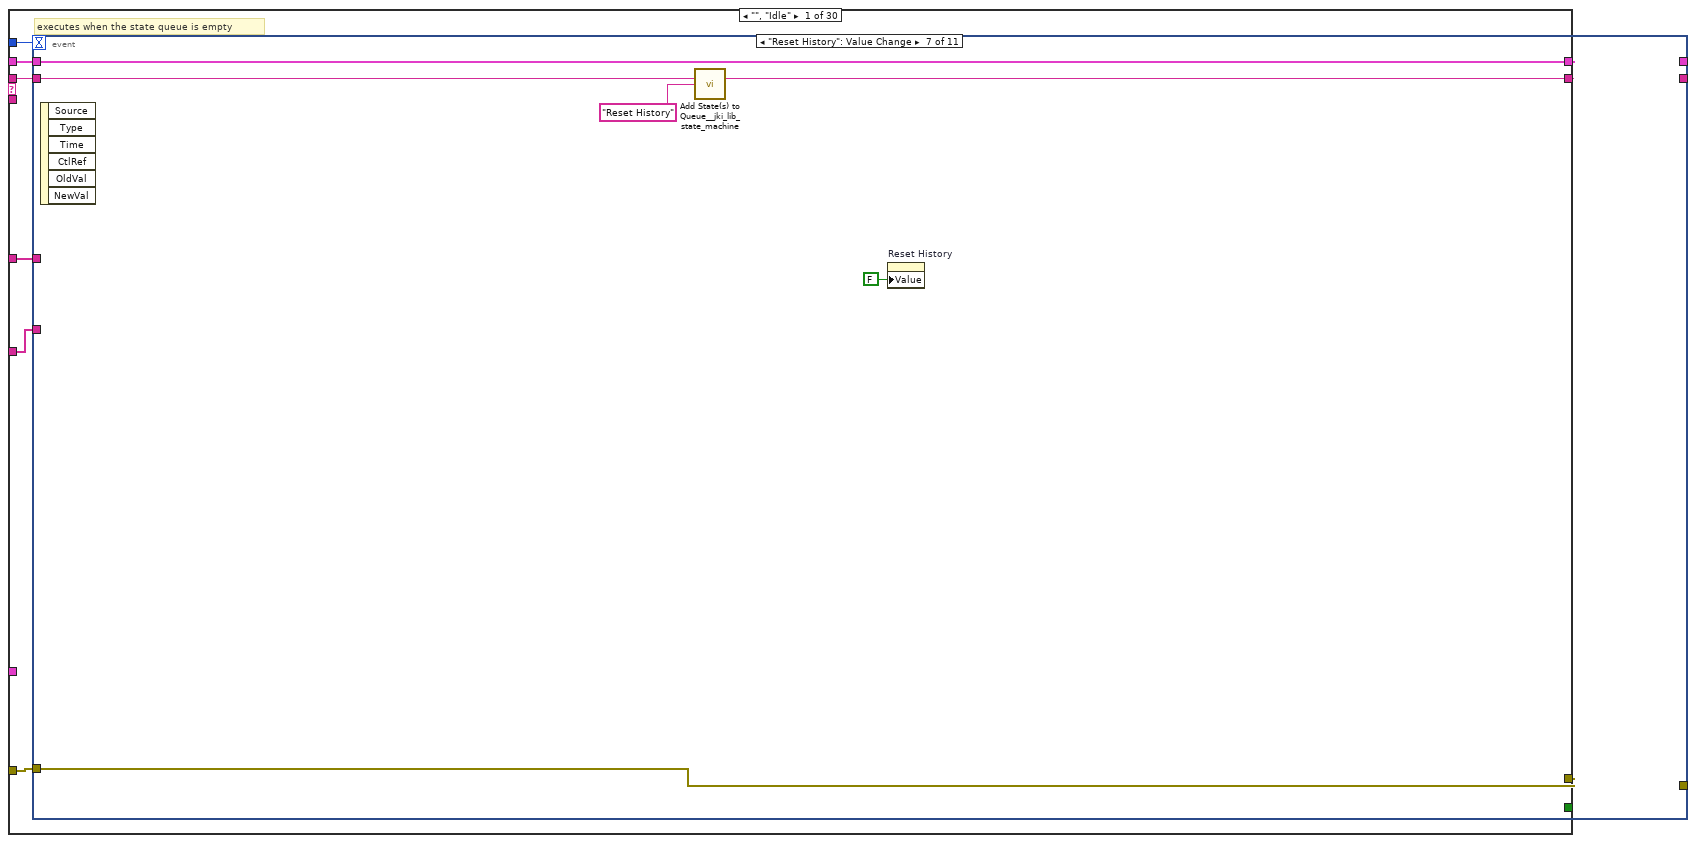
[diagram p3: hidden frame]
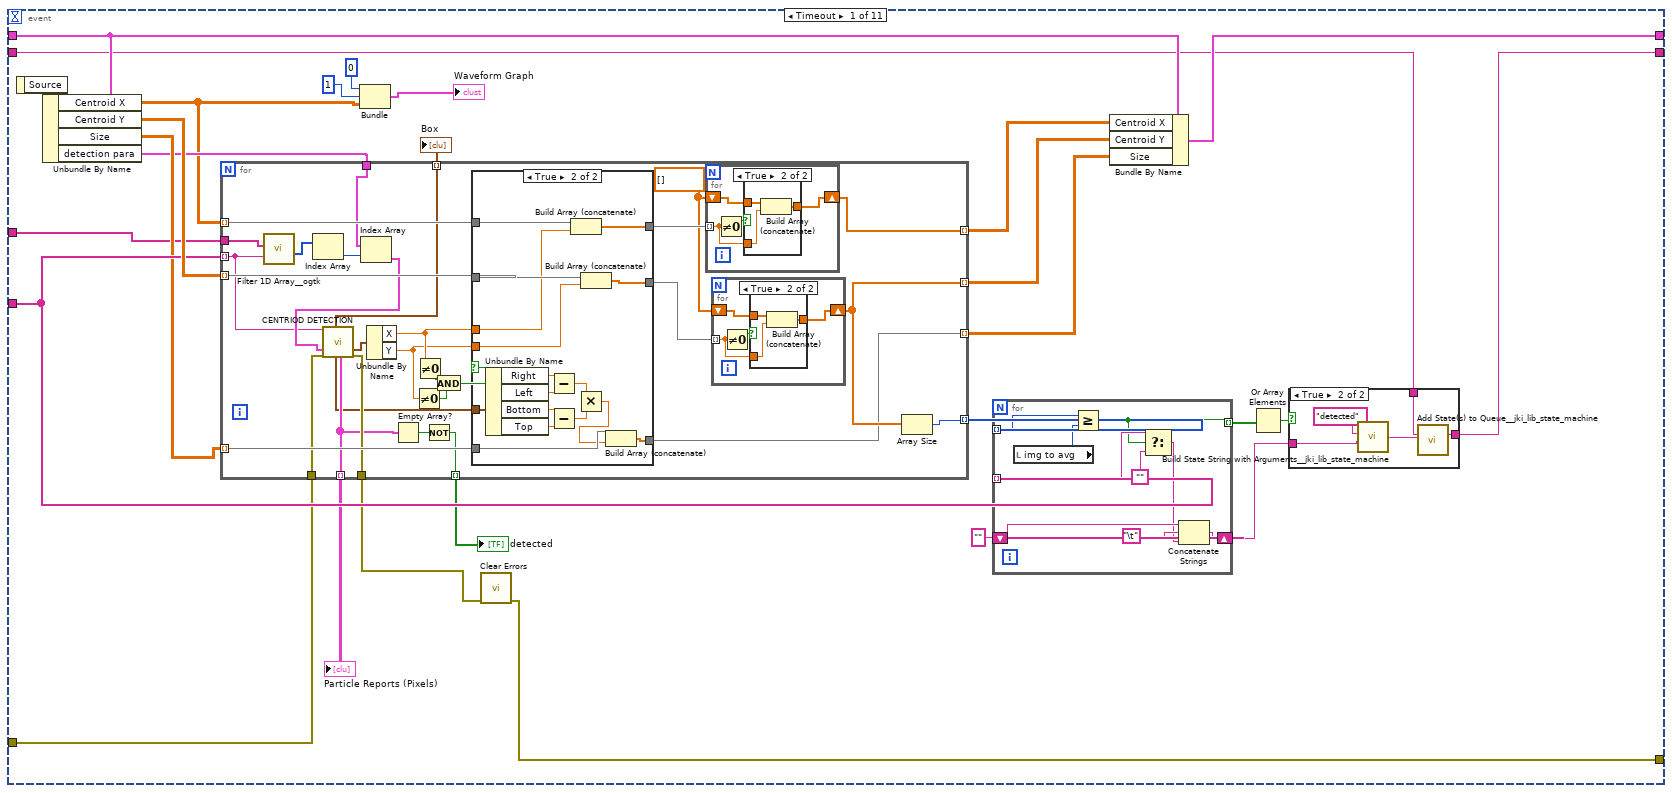
[diagram p4: hidden frame]
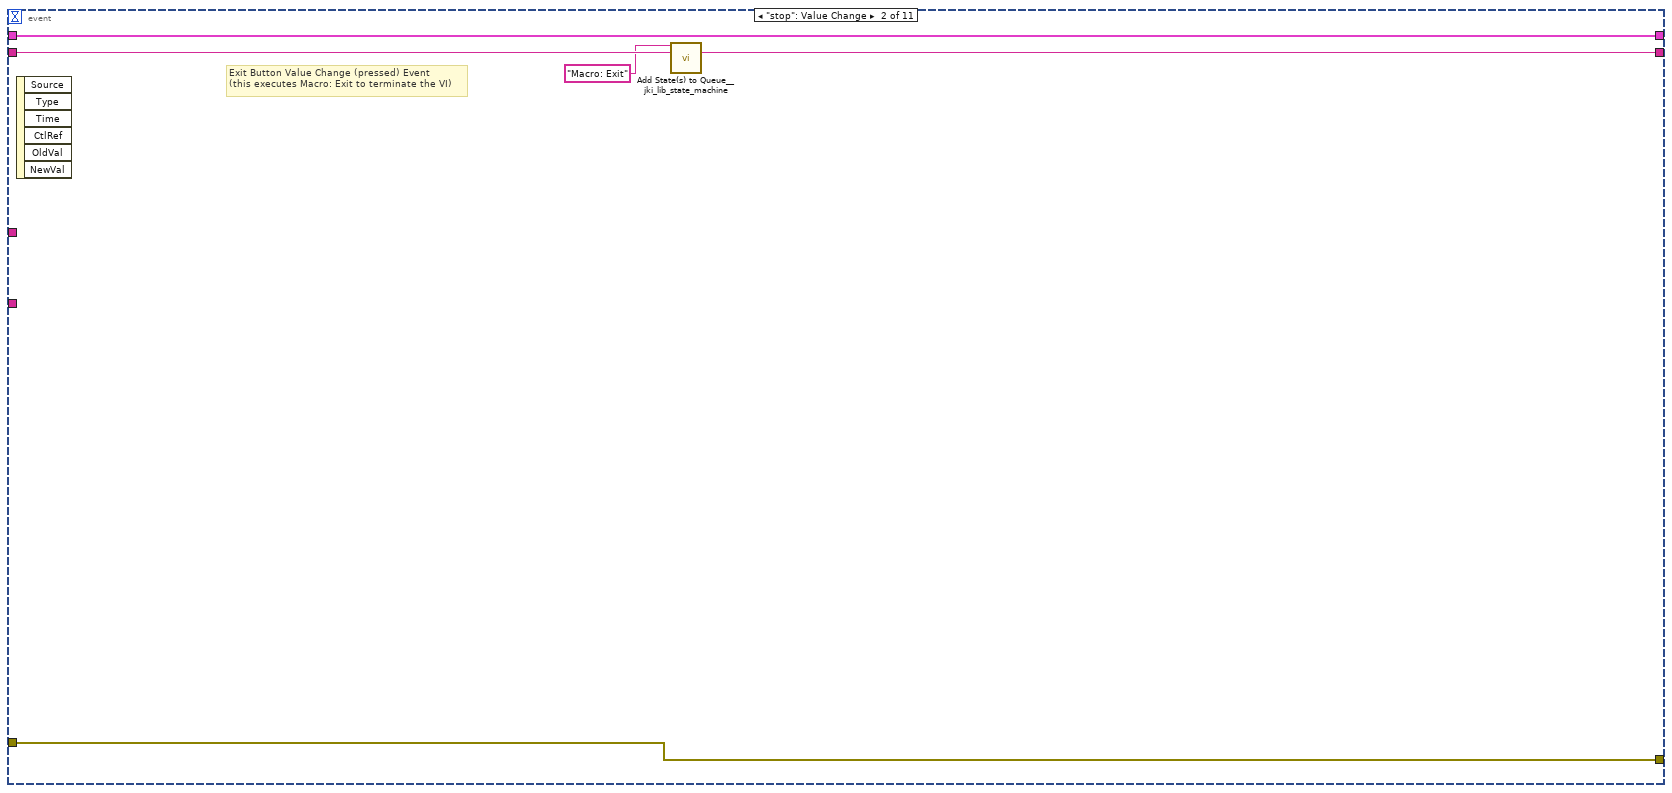
[diagram p9: hidden frame]
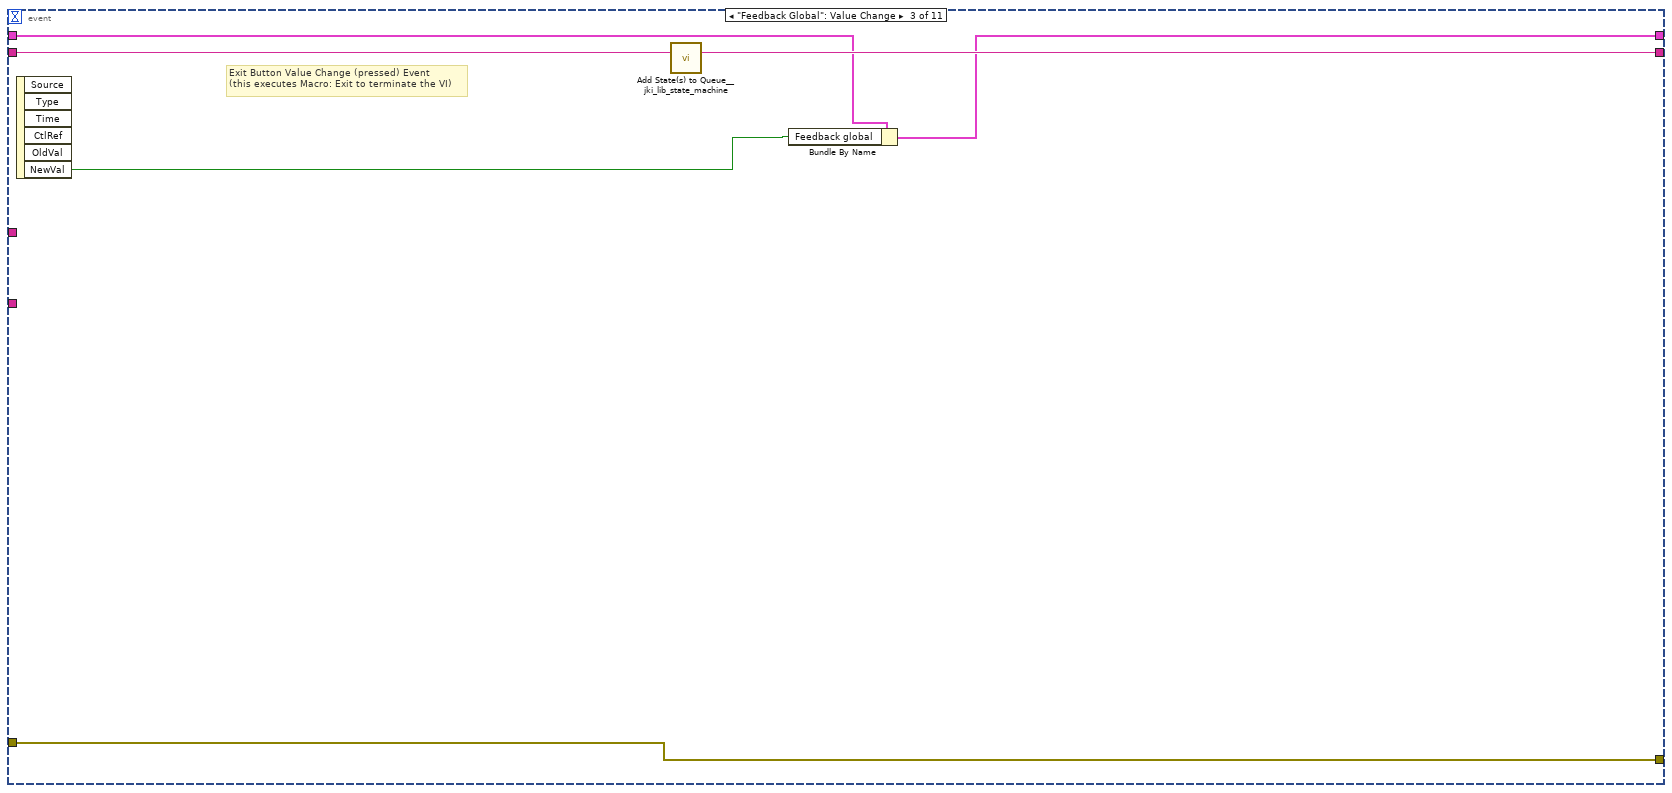
[diagram p10: hidden frame]
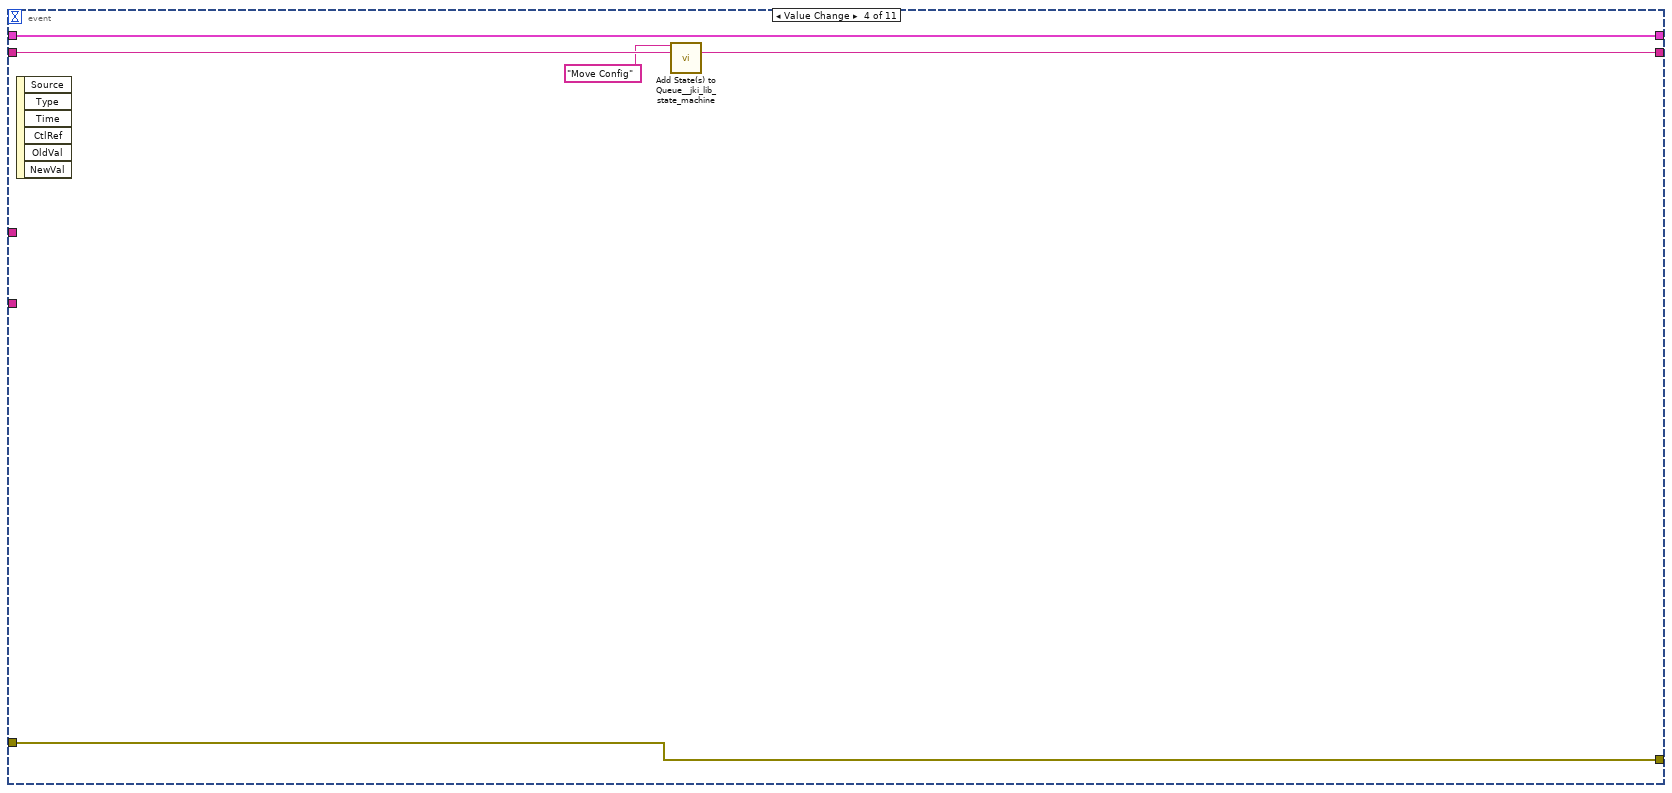
[diagram p11: hidden frame]
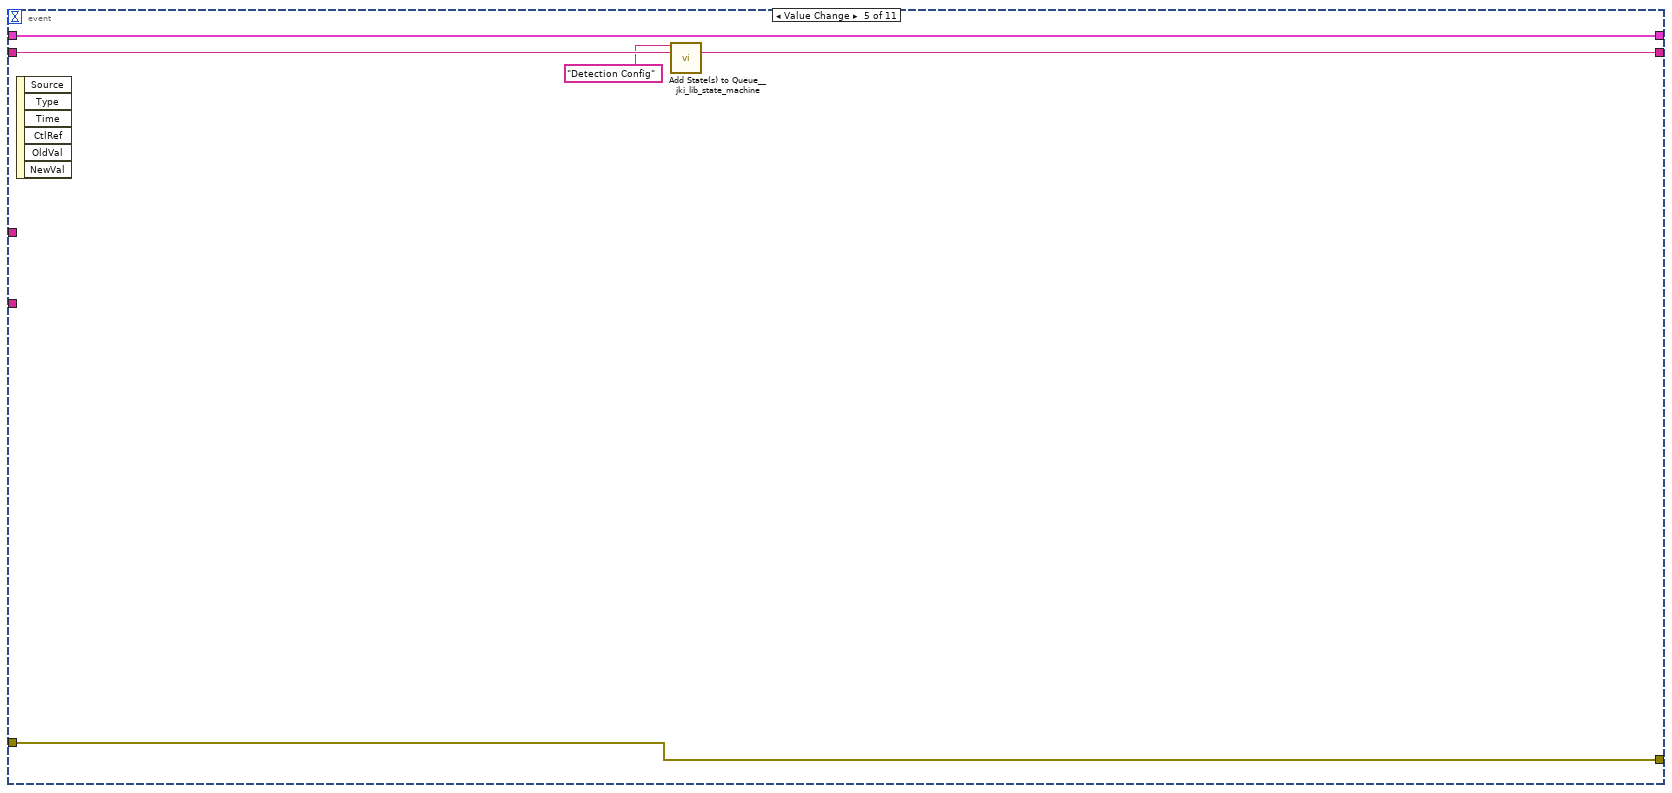
[diagram p12: hidden frame]
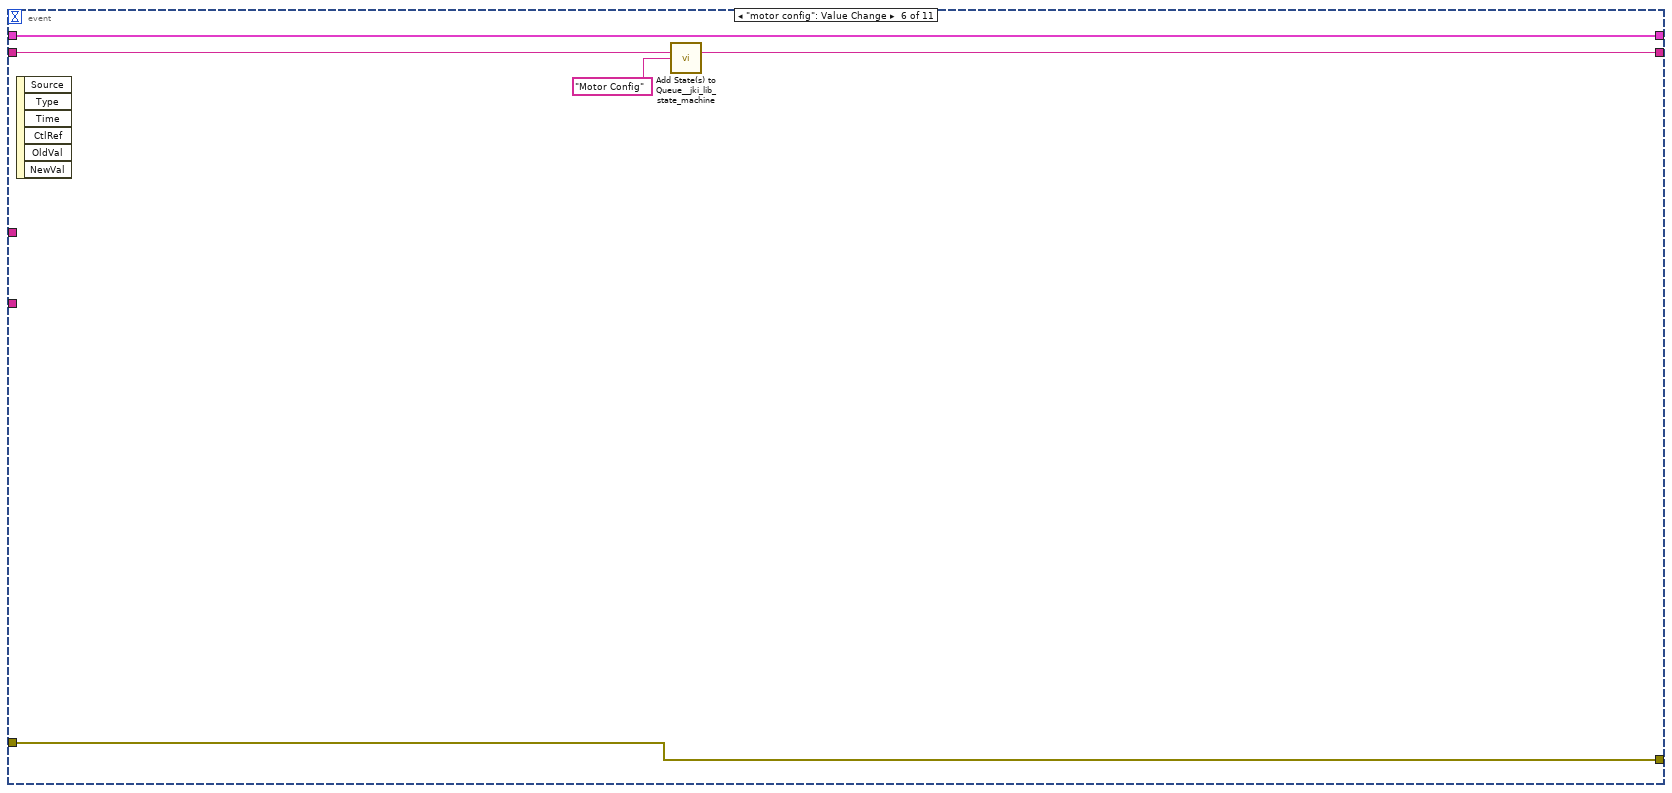
[diagram p13: hidden frame]
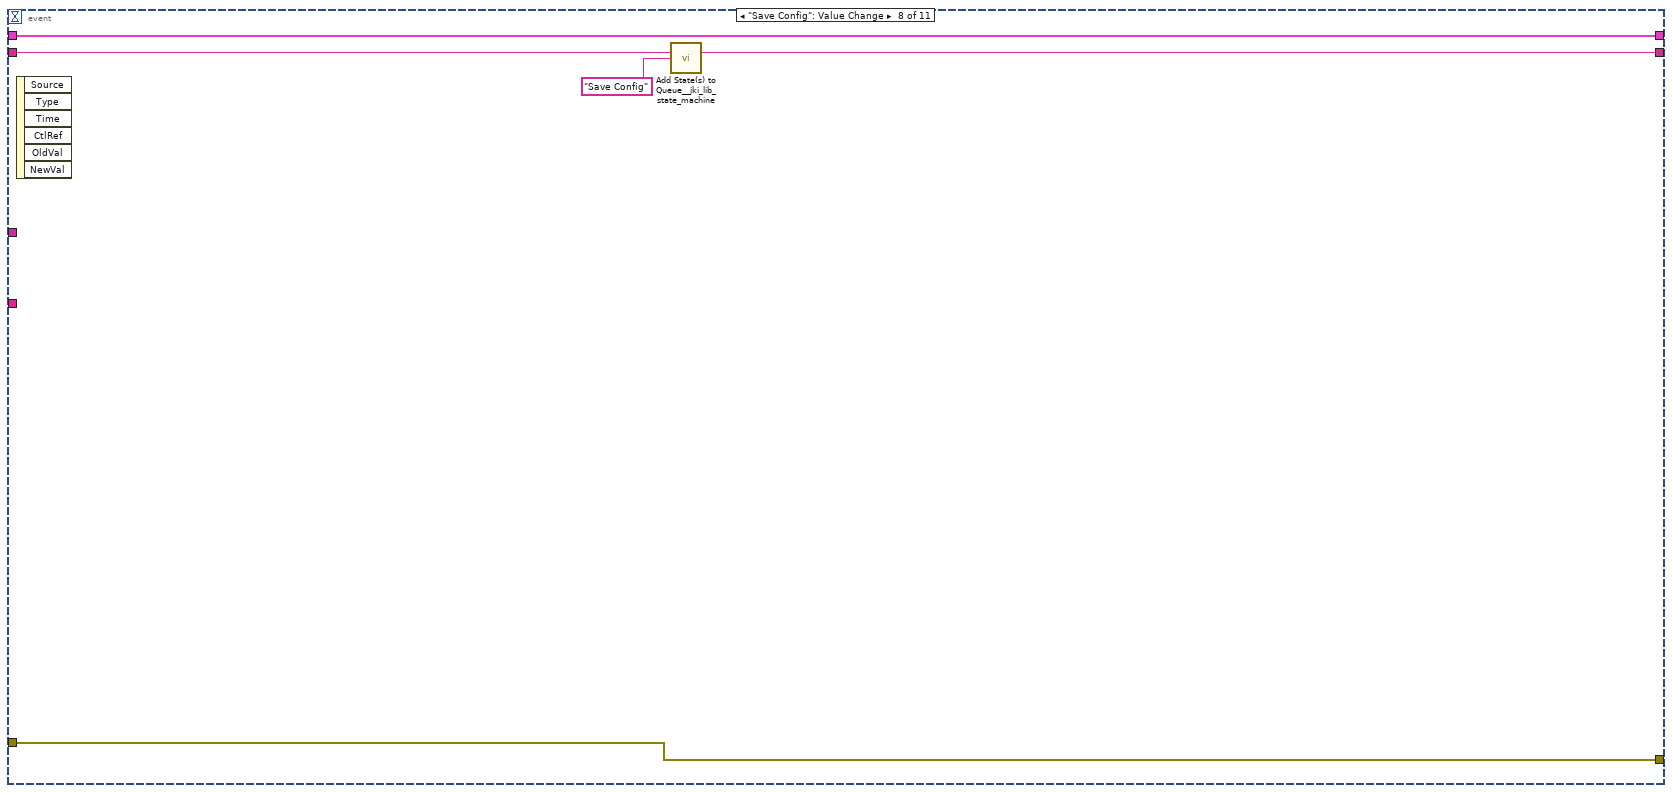
[diagram p14: hidden frame]
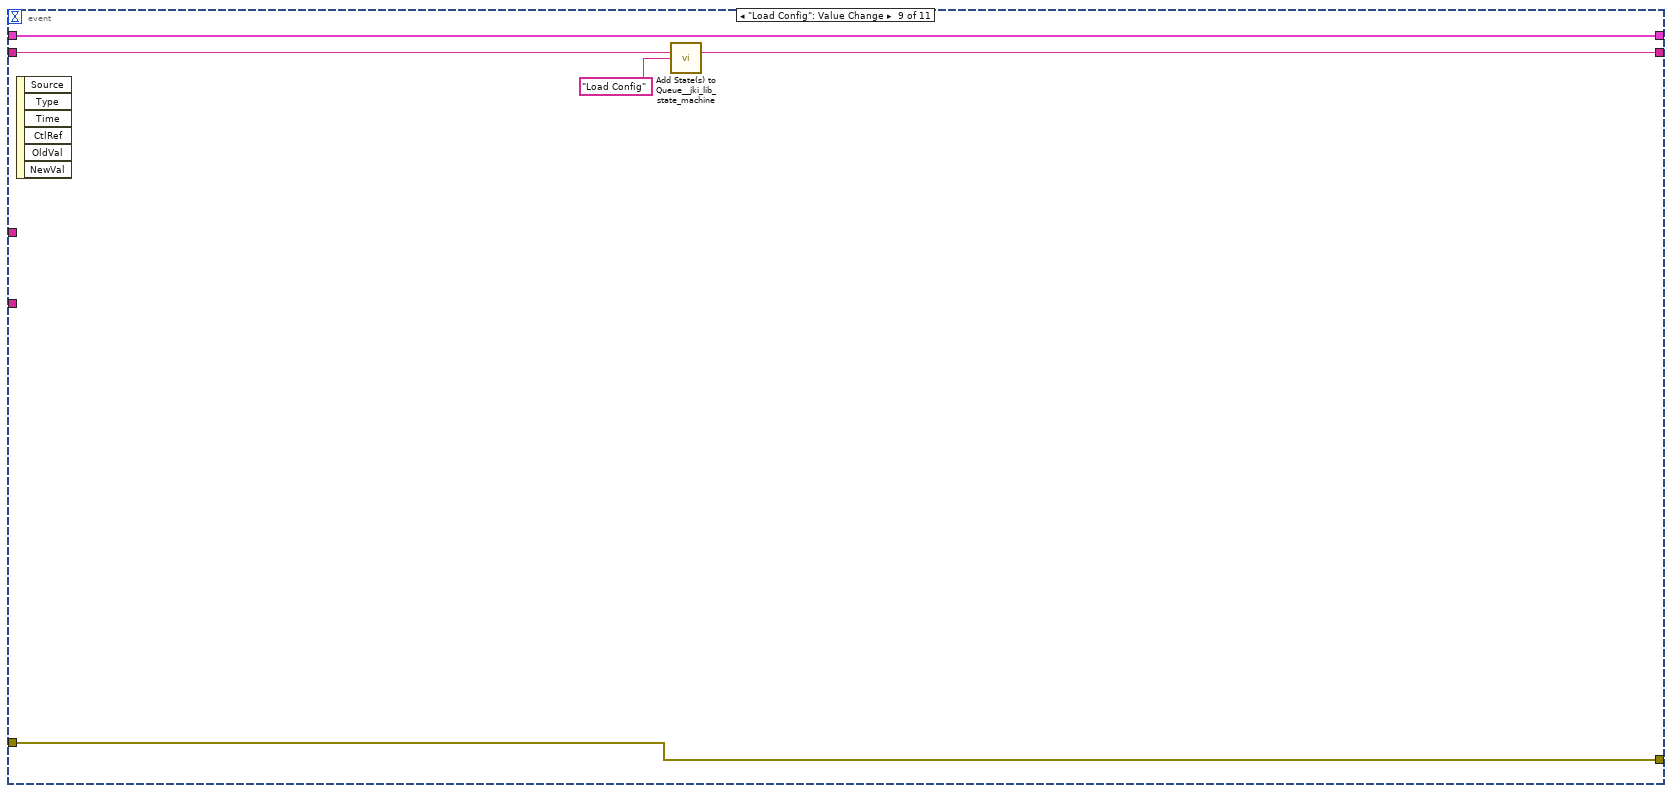
[diagram p15: hidden frame]
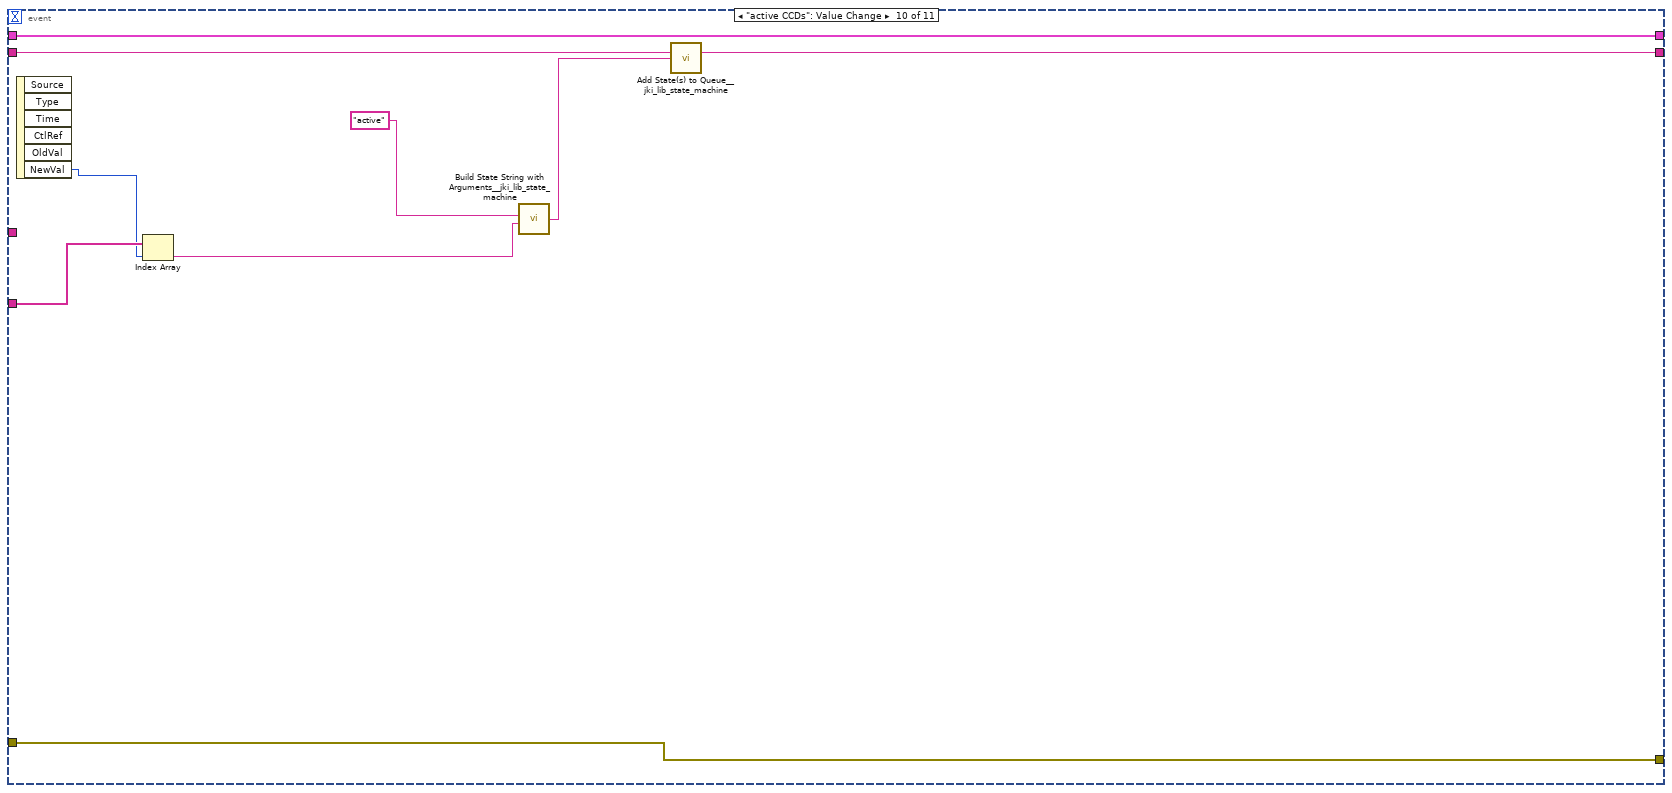
[diagram p16: hidden frame]
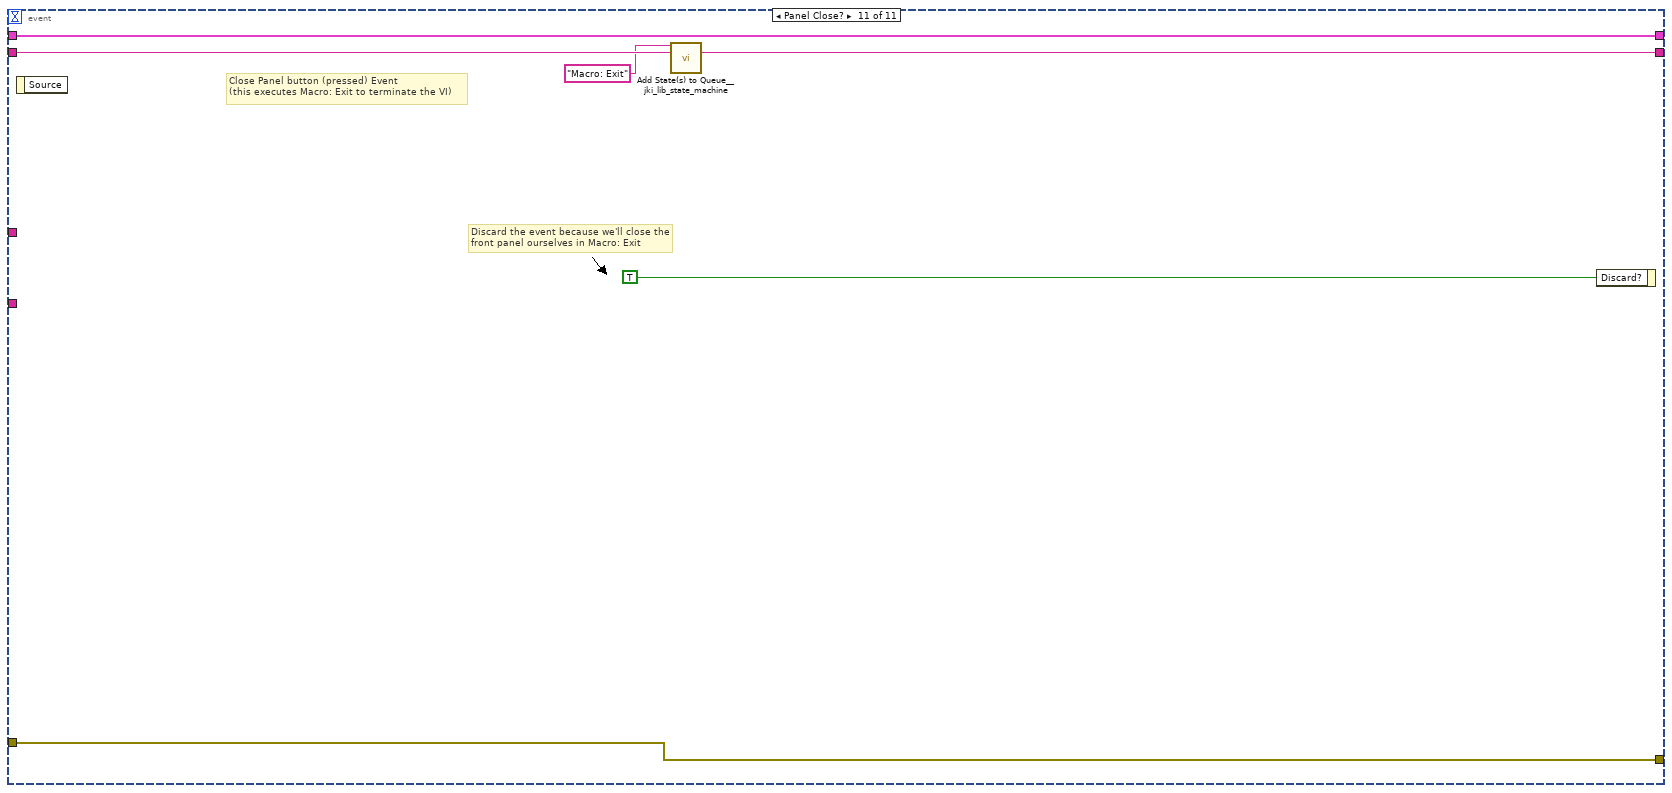
[diagram p17: hidden frame]
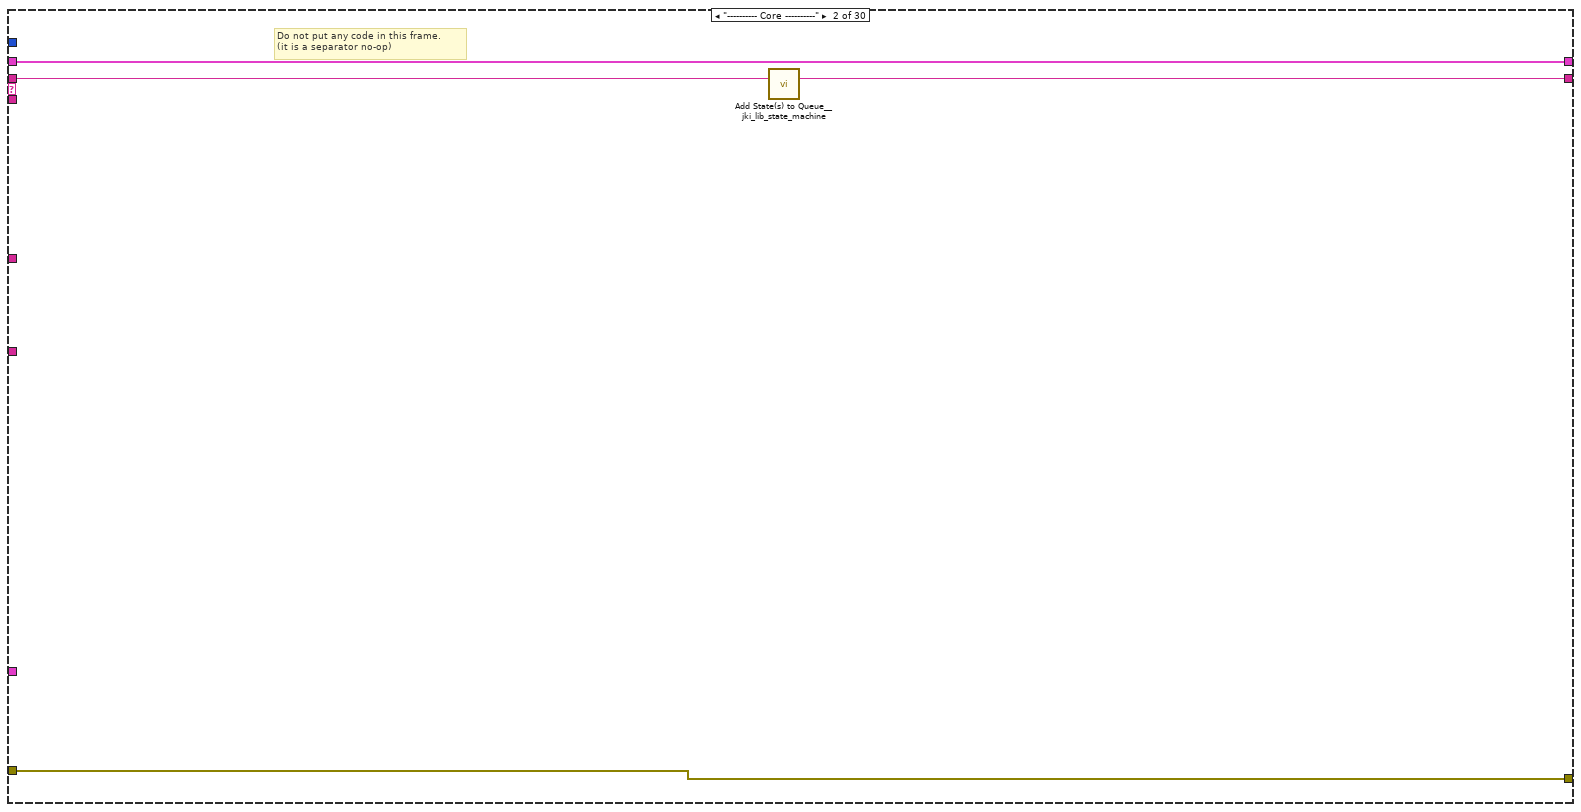
[diagram p18: hidden frame]
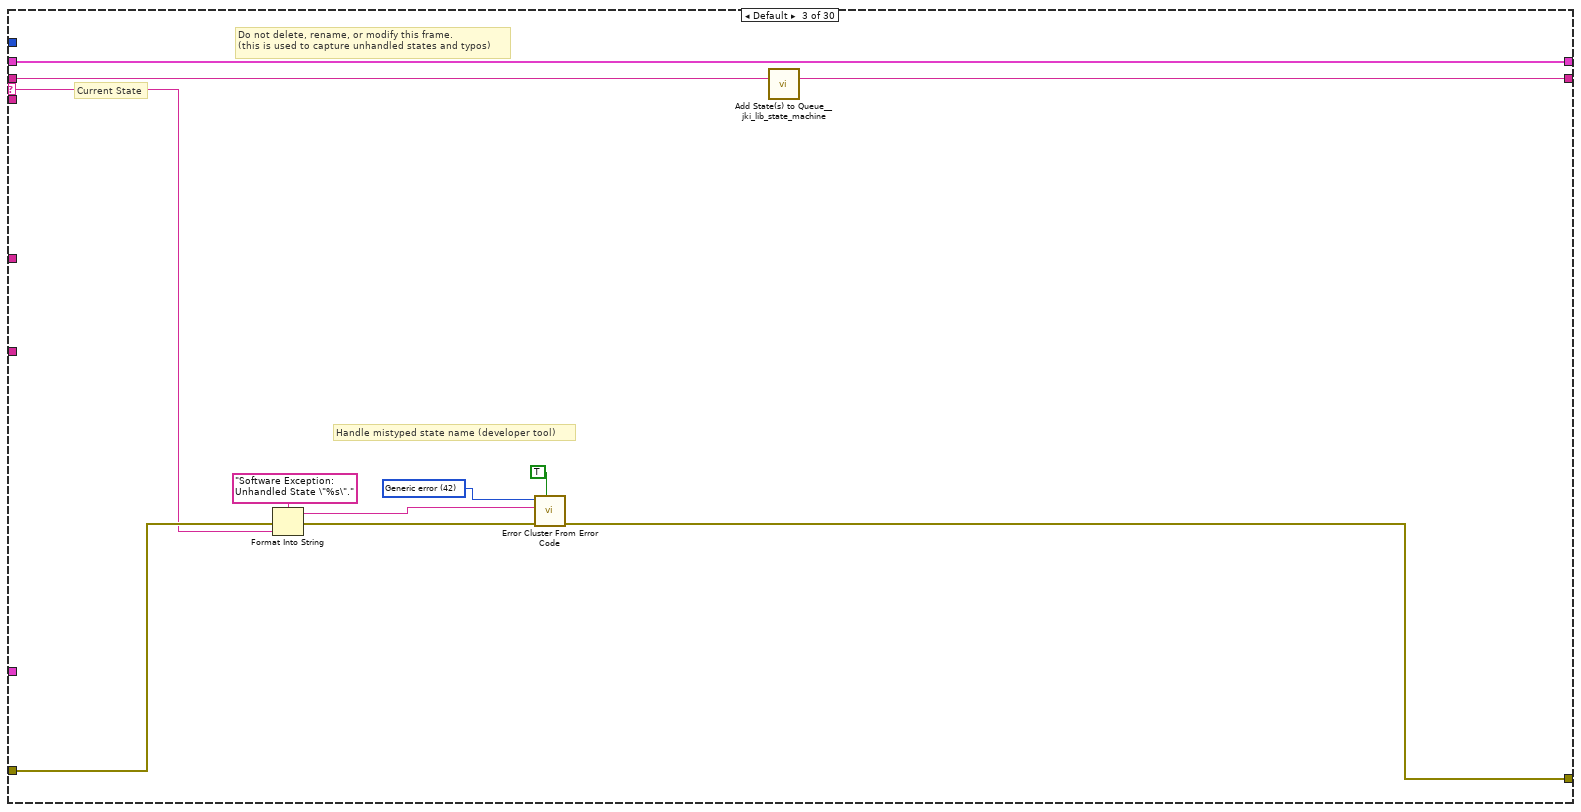
[diagram p19: hidden frame]
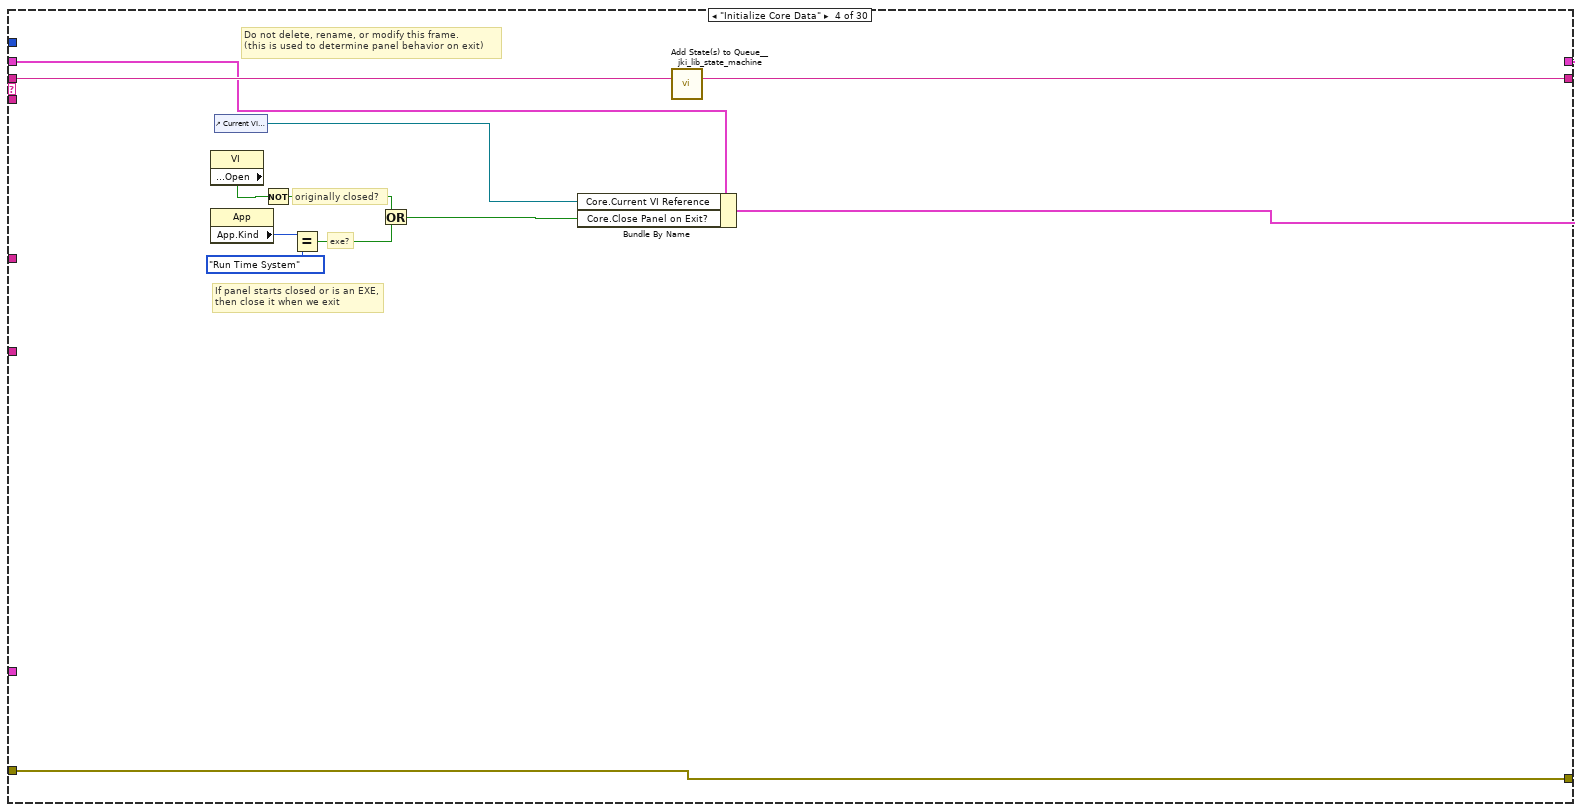
[diagram p20: hidden frame]
diagram:
  w62 = T13 1 items=["Grayscale (U8)", "Grayscale (I16)", "Grayscale (SGL)", "Complex (CSG)", "RGB (U32)", "HSL (U32)", "RGB (U64)", "Grayscale (U16)"] ("Image Type")
  # "NOT FOR YOU MOFO"
  n1 = call "getMotorNames.vi"("DeviceName"="GUIdevice 99") -> ("elements"=w28:string[])  [unwired: 10 in]
  n2 = control-ref of="Position.Axis 111::99"() -> (w132:refnum<vi>)
  n3 = control-ref of="Position.Axis 112::99"() -> (w131:refnum<vi>)
  n4 = control-ref of="Position.Axis 113::99"() -> (w130:refnum<vi>)
  n5 = control-ref of="Position.Axis 121::99"() -> (w129:refnum<vi>)
  n6 = control-ref of="Position.Axis 122::99"() -> (w128:refnum<vi>)
  n7 = control-ref of="Position.Axis 123::99"() -> (w127:refnum<vi>)
  n8 = control-ref of="Position.Axis 131::99"() -> (w126:refnum<vi>)
  n9 = control-ref of="Position.Axis 132::99"() -> (w125:refnum<vi>)
  n10 = control-ref of="Position.Axis 133::99"() -> (w124:refnum<vi>)
  n11 = control-ref of="Position.Axis 141::99"() -> (w123:refnum<vi>)
  n12 = control-ref of="Position.Axis 142::99"() -> (w122:refnum<vi>)
  n13 = control-ref of="Position.Axis 143::99"() -> (w121:refnum<vi>)
  n14 = control-ref of="Position.Axis 211::99"() -> (w120:refnum<vi>)
  n15 = control-ref of="Position.Axis 212::99"() -> (w119:refnum<vi>)
  n16 = control-ref of="Position.Axis 213::99"() -> (w118:refnum<vi>)
  n17 = control-ref of="Position.Axis 221::99"() -> (w117:refnum<vi>)
  n18 = control-ref of="Position.Axis 222::99"() -> (w116:refnum<vi>)
  n19 = control-ref of="Position.Axis 223::99"() -> (w115:refnum<vi>)
  n20 = control-ref of="Position.Axis 231::99"() -> (w114:refnum<vi>)
  n21 = control-ref of="Position.Axis 232::99"() -> (w113:refnum<vi>)
  n22 = control-ref of="Position.Axis 233::99"() -> (w112:refnum<vi>)
  n23 = control-ref of="Position.Axis 241::99"() -> (w111:refnum<vi>)
  n24 = control-ref of="Position.Axis 242::99"() -> (w110:refnum<vi>)
  n25 = control-ref of="Position.Axis 243::99"() -> (w109:refnum<vi>)
  n26 = control-ref of="Position.Axis 311::99"() -> (w108:refnum<vi>)
  n27 = control-ref of="Position.Axis 312::99"() -> (w107:refnum<vi>)
  n28 = control-ref of="Position.Axis 313::99"() -> (w106:refnum<vi>)
  n29 = control-ref of="Position.Axis 321::99"() -> (w105:refnum<vi>)
  n30 = control-ref of="Position.Axis 322::99"() -> (w104:refnum<vi>)
  n31 = control-ref of="Position.Axis 323::99"() -> (w103:refnum<vi>)
  n32 = control-ref of="Position.Axis 331::99"() -> (w102:refnum<vi>)
  n33 = control-ref of="Position.Axis 332::99"() -> (w101:refnum<vi>)
  n34 = control-ref of="Position.Axis 333::99"() -> (w100:refnum<vi>)
  n35 = control-ref of="Position.Axis 341::99"() -> (w99:refnum<vi>)
  n36 = control-ref of="Position.Axis 342::99"() -> (w98:refnum<vi>)
  n37 = control-ref of="Position.Axis 343::99"() -> (w97:refnum<vi>)
  n38 = control-ref of="Position.Axis 411::99"() -> (w96:refnum<vi>)
  n39 = control-ref of="Position.Axis 412::99"() -> (w95:refnum<vi>)
  n40 = control-ref of="Position.Axis 413::99"() -> (w94:refnum<vi>)
  n41 = control-ref of="Position.Axis 421::99"() -> (w93:refnum<vi>)
  n42 = control-ref of="Position.Axis 422::99"() -> (w92:refnum<vi>)
  n43 = control-ref of="Position.Axis 423::99"() -> (w91:refnum<vi>)
  n44 = control-ref of="Position.Axis 431::99"() -> (w90:refnum<vi>)
  n45 = control-ref of="Position.Axis 432::99"() -> (w89:refnum<vi>)
  n46 = control-ref of="Position.Axis 433::99"() -> (w88:refnum<vi>)
  n47 = control-ref of="Position.Axis 441::99"() -> (w87:refnum<vi>)
  n48 = control-ref of="Position.Axis 442::99"() -> (w86:refnum<vi>)
  n49 = control-ref of="Position.Axis 443::99"() -> (w85:refnum<vi>)
  n50 = control-ref of="Position.Axis 511::99"() -> (w84:refnum<vi>)
  n51 = control-ref of="Position.Axis 512::99"() -> (w83:refnum<vi>)
  n52 = control-ref of="Position.Axis 513::99"() -> (w82:refnum<vi>)
  n53 = control-ref of="Position.Axis 521::99"() -> (w81:refnum<vi>)
  n54 = control-ref of="Position.Axis 522::99"() -> (w80:refnum<vi>)
  n55 = control-ref of="Position.Axis 523::99"() -> (w79:refnum<vi>)
  n56 = control-ref of="Position.Axis 531::99"() -> (w78:refnum<vi>)
  n57 = control-ref of="Position.Axis 532::99"() -> (w77:refnum<vi>)
  n58 = control-ref of="Position.Axis 533::99"() -> (w76:refnum<vi>)
  n59 = control-ref of="Position.Axis 541::99"() -> (w75:refnum<vi>)
  n60 = control-ref of="Position.Axis 542::99"() -> (w74:refnum<vi>)
  n61 = control-ref of="Position.Axis 543::99"() -> (w73:refnum<vi>)
  n62 = property on="Motor CCD 1" class="Ring (strict)"("Strings []"=w28) -> ()  [unwired: 2 in, 2 out]
  n63 = property on="Motor CCD 2" class="Ring (strict)"("Strings []"=w28) -> ()  [unwired: 2 in, 2 out]
  n64 = property on="Motor CCD 3" class="Ring (strict)"("Strings []"=w28) -> ()  [unwired: 2 in, 2 out]
  n65 = property on="Motor CCD 4" class="Ring (strict)"("Strings []"=w28) -> ()  [unwired: 2 in, 2 out]
  n66 = property on="Motor CCD 5" class="Ring (strict)"("Strings []"=w28) -> ()  [unwired: 2 in, 2 out]
  n67 = property on="Motor CCD 6" class="Ring (strict)"("Strings []"=w28) -> ()  [unwired: 2 in, 2 out]
  n68 = property on="Motor CCD 7" class="Ring (strict)"("Strings []"=w28) -> ()  [unwired: 2 in, 2 out]
  n69 = property on="Motor CCD 8" class="Ring (strict)"("Strings []"=w28) -> ()  [unwired: 2 in, 2 out]
  n70 = property on="Motor CCD 9" class="Ring (strict)"("Strings []"=w28) -> ()  [unwired: 2 in, 2 out]
  n71 = property on="Motor CCD 10" class="Ring (strict)"("Strings []"=w28) -> ()  [unwired: 2 in, 2 out]
  n72 = property on="Motor CCD 11" class="Ring (strict)"("Strings []"=w28) -> ()  [unwired: 2 in, 2 out]
  n73 = property on="Motor CCD 12" class="Ring (strict)"("Strings []"=w28) -> ()  [unwired: 2 in, 2 out]
  n74 = Build Array(w132, w131, w130, w129, w128, w127, w126, w125, w124, w123, w122, w121, w120, w119, w118, w117, w116, w115, w114, w113, w112, w111, w110, w109, w108, w107, w106, w105, w104, w103, w102, w101, w100, w99, w98, w97, w96, w95, w94, w93, w92, w91, w90, w89, w88, w87, w86, w85, w84, w83, w82, w81, w80, w79, w78, w77, w76, w75, w74, w73) -> (→"motor refs":refnum<vi>[])
  n75 = control-ref of="Target.X::1"() -> (w52:refnum<vi>)
  n76 = control-ref of="Target.Y::1"() -> (w51:refnum<vi>)
  n77 = control-ref of="Target.X::2"() -> (w50:refnum<vi>)
  n78 = control-ref of="Target.Y::2"() -> (w49:refnum<vi>)
  n79 = control-ref of="Target.X::3"() -> (w48:refnum<vi>)
  n80 = control-ref of="Target.Y::3"() -> (w47:refnum<vi>)
  n81 = control-ref of="Target.X::4"() -> (w46:refnum<vi>)
  n82 = control-ref of="Target.Y::4"() -> (w45:refnum<vi>)
  n83 = control-ref of="Target.X::5"() -> (w44:refnum<vi>)
  n84 = control-ref of="Target.Y::5"() -> (w43:refnum<vi>)
  n85 = control-ref of="Target.X::6"() -> (w42:refnum<vi>)
  n86 = control-ref of="Target.Y::6"() -> (w41:refnum<vi>)
  n87 = control-ref of="Target.X::7"() -> (w40:refnum<vi>)
  n88 = control-ref of="Target.Y::7"() -> (w39:refnum<vi>)
  n89 = control-ref of="Target.X::8"() -> (w38:refnum<vi>)
  n90 = control-ref of="Target.Y::8"() -> (w37:refnum<vi>)
  n91 = for {
    N: 1 -> [_]
    shift-right: [w154] -> w53
    shift-left: timestamp[][] [] ("Time") -> [w156]
    n92 = for {
      N: 12 -> [_]
      tunnel: w156 -> [w159] mode=indexing
      tunnel: [w157] -> w154 mode=indexing
      n93 = Get Date/Time In Seconds() -> (seconds since 1Jan1904=w158:timestamp)
      n94 = Build Array (concatenate)(w159, w158) -> (w157:timestamp[])
    }
  }
  n95 = Bundle("Target.X::1"="Target.X::1", "Target.Y::1"="Target.Y::1") -> (w11:cluster{"Target.X::1":dbl, "Target.Y::1":dbl})  [unwired: 1 in]
  n96 = Bundle("Target.X::2"="Target.X::2", "Target.Y::2"="Target.Y::2") -> (w10:cluster{"Target.X::2":dbl, "Target.Y::2":dbl})  [unwired: 1 in]
  n97 = Bundle("Target.X::3"="Target.X::3", "Target.Y::3"="Target.Y::3") -> (w9:cluster{"Target.X::3":dbl, "Target.Y::3":dbl})  [unwired: 1 in]
  n98 = Bundle("Target.X::4"="Target.X::4", "Target.Y::4"="Target.Y::4") -> (w8:cluster{"Target.X::4":dbl, "Target.Y::4":dbl})  [unwired: 1 in]
  n99 = Bundle("Target.X::5"="Target.X::5", "Target.Y::5"="Target.Y::5") -> (w7:cluster{"Target.X::5":dbl, "Target.Y::5":dbl})  [unwired: 1 in]
  n100 = Bundle("Target.X::6"="Target.X::6", "Target.Y::6"="Target.Y::6") -> (w6:cluster{"Target.X::6":dbl, "Target.Y::6":dbl})  [unwired: 1 in]
  n101 = Bundle("Target.X::7"="Target.X::7", "Target.Y::7"="Target.Y::7") -> (w5:cluster{"Target.X::7":dbl, "Target.Y::7":dbl})  [unwired: 1 in]
  n102 = Bundle("Target.X::8"="Target.X::8", "Target.Y::8"="Target.Y::8") -> (w2:cluster{"Target.X::8":dbl, "Target.Y::8":dbl})  [unwired: 1 in]
  n103 = Bundle("Target.X::1"=w52, "Target.Y::1"=w51) -> (w36:T15)  [unwired: 1 in]
  n104 = Bundle("Target.X::2"=w50, "Target.Y::2"=w49) -> (w35:T16)  [unwired: 1 in]
  n105 = Bundle("Target.X::3"=w48, "Target.Y::3"=w47) -> (w34:T17)  [unwired: 1 in]
  n106 = Bundle("Target.X::4"=w46, "Target.Y::4"=w45) -> (w1:T18)  [unwired: 1 in]
  n107 = Bundle("Target.X::5"=w44, "Target.Y::5"=w43) -> (w33:T19)  [unwired: 1 in]
  n108 = Bundle("Target.X::6"=w42, "Target.Y::6"=w41) -> (w32:T20)  [unwired: 1 in]
  n109 = Bundle("Target.X::7"=w40, "Target.Y::7"=w39) -> (w31:T21)  [unwired: 1 in]
  n110 = Bundle("Target.X::8"=w38, "Target.Y::8"=w37) -> (w30:T22)  [unwired: 1 in]
  n111 = Build Array(w36, w35, w34, w1, w33, w32, w31, w30) -> (w29:T23)
  n112 = Build Array(w11, w10, w9, w8, w7, w6, w5, w2) -> ()  [unwired: 1 out]
  n113 = property on="Time" class="Arr (strict)"("Value"=w53) -> ()  [unwired: 2 in, 2 out]
  n114 = call "IMAQ Create"("Image Name"="GUIdevice 8", "Image Type"=w62) -> ("New Image"=→"image::8":T5)  [unwired: 3 in, 1 out]
  n115 = call "IMAQ Create"("Image Name"="GUIdevice 6", "Image Type"=w62) -> ("New Image"=→"image::6":T5)  [unwired: 3 in, 1 out]
  n116 = call "IMAQ Create"("Image Name"="GUIdevice 7", "Image Type"=w62) -> ("New Image"=→"image::7":T5)  [unwired: 3 in, 1 out]
  n117 = call "IMAQ Create"("Image Name"="GUIdevice 2") -> ("New Image"=→"image::2":T5)  [unwired: 4 in, 1 out]
  n118 = call "IMAQ Create"("Image Name"="GUIdevice 4", "Image Type"=w62) -> ("New Image"=→"image::4":T5)  [unwired: 3 in, 1 out]
  n119 = call "IMAQ Create"("Image Name"="GUIdevice 1", "Image Type"=w62) -> ("New Image"=→"image::1":T5)  [unwired: 3 in, 1 out]
  n120 = call "IMAQ Create"("Image Name"="GUIdevice 3", "Image Type"=w62) -> ("New Image"=→"image::3":T5)  [unwired: 3 in, 1 out]
  n121 = call "IMAQ Create"("Image Name"="GUIdevice 5", "Image Type"=w62) -> ("New Image"=→"image::5":T5)  [unwired: 3 in, 1 out]
  n122 = Build Array("GUIdevice 1", "GUIdevice 2", "GUIdevice 3", "GUIdevice 4", "GUIdevice 5", "GUIdevice 6", "GUIdevice 7", "GUIdevice 8") -> (w60:string[])
  n123 = property on="image::8" class="ImageControl"("Caption.Text"="GUIdevice 8") -> ()  [unwired: 2 in, 2 out]
  n124 = property on="image::1" class="ImageControl"("Caption.Text"="GUIdevice 1") -> ()  [unwired: 2 in, 2 out]
  n125 = property on="image::2" class="ImageControl"("Caption.Text"="GUIdevice 2") -> ()  [unwired: 2 in, 2 out]
  n126 = property on="image::3" class="ImageControl"("Caption.Text"="GUIdevice 3") -> ()  [unwired: 2 in, 2 out]
  n127 = property on="image::4" class="ImageControl"("Caption.Text"="GUIdevice 4") -> ()  [unwired: 2 in, 2 out]
  n128 = property on="image::5" class="ImageControl"("Caption.Text"="GUIdevice 5") -> ()  [unwired: 2 in, 2 out]
  n129 = property on="image::6" class="ImageControl"("Caption.Text"="GUIdevice 6") -> ()  [unwired: 2 in, 2 out]
  n130 = property on="image::7" class="ImageControl"("Caption.Text"="GUIdevice 7") -> ()  [unwired: 2 in, 2 out]
  n131 = Array To Cluster(array=w60) -> (cluster=→"CCDs 2":T4)
  n132 = property on="CCDs" class="Ring (strict)"("Strings []"=w60) -> ()  [unwired: 2 in, 2 out]
  n133 = Empty String/Path?(string/path=w60) -> (empty?=w135:bool[])
  n134 = for {
    tunnel: w135 -> [w162] mode=indexing
    shift-right: [w160] -> w133
    shift-left: w60 -> [w161]
    n135 = case shown="True" w162 {
      tunnel: w161 -> [w163 w165]
      tunnel: [w163 w164] -> w160
      frame False {
      }
      frame True {
        n136 = Delete From Array(array=w165) -> (array with subset deleted=w164:string[])  [unwired: 2 in, 1 out]
      }
    }
  }
  n137 = Array Size(array=w133) -> (size(s)=w136:i32)
  n138 = property on="Feedback Global" class="Bool (strict)"("Value"=FALSE ("Feedback Global")) -> ()  [unwired: 2 in, 2 out]
  n139 = Initialize Array(0.0 ("element"), w136, 0 ("dimension size")) -> (w27:dbl[][])
  n140 = local write "Mean Centroid X"(w27) -> ()
  n141 = local write "Mean Centroid Y"(w27) -> ()
  n142 = local write "Offset Y stats"(w27) -> ()
  n143 = property on="active CCDs" class="LstBox (strict)"("Item Names"=w133) -> ()  [unwired: 2 in, 2 out]
  n144 = local write "Offset X stats"(w27) -> ()
  n145 = local write "Centroid X"(w27) -> ()
  n146 = local write "Centroid Y"(w27) -> ()
  n147 = local write "Mean Size"(w27) -> ()
  n148 = local write "Offset X"(w27) -> ()
  n149 = local write "Offset Y"(w27) -> ()
  n150 = local write "Size"(w27) -> ()
  n151 = Create User Event(user event datatype=T14 {"EventEnum"=enum."new data", "Device name"="Device name"} ("New Event")) -> (user event=w147:refnum<user-event>, error out=w149:errorcluster)  [unwired: 1 in]
  "tcp data event" <- w147
  n152 = call <vilib>:"Add State(s) to Queue__jki_lib_state_machine.vi"("State(s) in (\"\")"="Macro: Initialize") -> ("States Out"=w139:string)  [unwired: 14 in]
  n153 = while "JKI - String-Based Queued State Machine (Basic) v1.0" {
    shift-right: [w174] -> _
    shift-left: _ -> [w173]
    shift-right: [w177] -> w57
    shift-left: _ -> [w172]
    shift-right: [w176] -> _
    shift-left: w139 -> [w178]
    tunnel: w133 -> [w167]
    tunnel: w29 -> [w170]
    tunnel: w60 -> [w168]
    tunnel: [w168] -> w58
    tunnel: w29 -> [w169]
    stop <- w175 stop-if-true
    n154 = call <vilib>:"Parse State Queue__jki_lib_state_machine.vi"("State Queue"=w178, "Error In (no error)"=w172) -> ("Remaining States"=w180:string, "Current State"=w181:string, "Arguments"=w179:string)  [unwired: 11 in]
    n155 = case shown="\"active\"" w181 {
      selector: w181 -> [_ _ w373 _ _ _ _ _ _ _ _ _ _ _ _ _ _ _ _ _ _ _ _ _ _ _ _ _ _ _]
      tunnel: w180 -> [w206 w372 w377 w395 w401 w406 w410 w432 w438 w442 w446 w452 w463 w487 w492 w502 w506 w554 w649 w742 w828 w892 w898 w916 w936 w943 w956 w965 w974 w996]
      tunnel: w179 -> [_ _ _ _ _ _ _ _ _ _ _ w447 w458 _ _ _ _ w550 _ w735 w821 _ _ _ _ _ w953 _ _ _]
      tunnel: w173 -> [w204 w369 w375 w385 w398 w404 w407 _ w433 w439 w444 w450 w457 w484 w489 w494 w503 w536 w647 w734 w820 w889 w894 w914 w918 w940 w948 w958 w970 w987]
      tunnel: [w203 w370 w379 w393 errorcluster {"status"=FALSE, "code"=0, "source"=""} ("error out") w403 w408 w430 w435 w440 w443 w448 w460 w485 w490 w500 w504 w552 w661 w740 w826 w890 w896 w905 w928 w941 w954 w963 w972 w994] -> w177
      tunnel: w172 -> [w202 w370 w378 w393 w397 w403 w408 w430 w436 w440 w443 w449 w461 w485 w490 w500 w504 w552 w661 w740 w826 w890 w896 w906 w929 w941 w954 w963 w972 w994]
      tunnel: [w205 w371 w376 w394 w400 w405 w409 w431 w437 w441 w445 w451 w462 w486 w491 w501 w505 w553 w662 w741 w827 w891 w897 w915 w935 w942 w955 w964 w973 w995] -> w176
      tunnel: [_ _ _ _ _ TRUE _ _ _ _ _ _ _ _ _ _ _ _ _ _ _ _ _ _ _ _ _ _ _ _] -> w175
      tunnel: [w201 w369 w375 w384 w398 w404 w407 w425 w433 w439 w444 w450 w457 w484 w489 w494 w503 w542 w647 w734 w820 w889 w893 w914 w917 w939 w947 w957 w969 w986] -> w174
      tunnel: "updat speed [ms]" -> [w200 _ _ _ _ _ _ _ _ _ _ _ _ _ _ _ _ _ _ _ _ _ _ _ _ _ _ _ _ _]
      tunnel: w167 -> [w199 _ _ _ _ _ _ _ _ _ _ _ _ _ _ _ _ w547 w654 _ _ _ _ _ _ _ _ _ _ _]
      tunnel: w170 -> [_ _ _ _ _ _ _ _ _ _ _ _ _ _ _ _ _ w537 _ _ _ _ _ _ _ _ _ _ _ _]
      tunnel: w168 -> [w198 _ _ _ _ _ _ _ _ _ _ _ _ _ _ _ _ _ _ w739 w825 _ _ _ _ _ w949 _ _ _]
      frame "", "Idle" {
        # "executes when the state queue is empty"
        n156 = event shown="[6] \"Reset History\": Value Change" {
          selector: _ -> [_ _ _ _ _ _ _ _ _ _ _]
          dyn-events: _ -> [_ _ _ _ _ _ _ _ _ _ _]
          timeout: w200 -> [_ _ _ _ _ _ _ _ _ _ _]
          tunnel: w206 -> [w222 w316 w322 w327 w332 w337 w343 w348 w353 w362 w368]
          tunnel: [w221 w315 w321 w326 w331 w336 w342 w347 w352 w361 w367] -> w205
          tunnel: w204 -> [w233 w313 w318 w324 w329 w334 w340 w345 w350 w359 w365]
          tunnel: [w216 w314 w320 w325 w330 w335 w341 w346 w351 w360 w366] -> w203
          tunnel: w202 -> [w217 w314 w320 w325 w330 w335 w341 w346 w351 w360 w366]
          tunnel: [w231 w313 w317 w324 w329 w334 w340 w345 w350 w359 w365] -> w201
          tunnel: w199 -> [w227 _ _ _ _ _ _ _ _ w358 _]
          tunnel: w198 -> [w215 _ _ _ _ _ _ _ _ _ _]
          event Timeout {
            n157 = event-data() -> ()  [unwired: 1 in, 1 out]
            n158 = Unbundle By Name(w233) -> ("Centroid X"=w211:dbl[][], "Centroid Y"=w230:dbl[][], "Size"=w220:dbl[][], "detection para"=w214:T6[])
            n159 = for {
              tunnel: w227 -> [w250] mode=indexing
              tunnel: [w266] -> w229 mode=indexing
              tunnel: [w263] -> w232 mode=indexing
              tunnel: [w271] -> w228 mode=indexing
              tunnel: w211 -> [w270] mode=indexing
              tunnel: w230 -> [w269] mode=indexing
              tunnel: w220 -> [w262] mode=indexing
              tunnel: [w261] -> w219 mode=indexing
              tunnel: [w260] -> w218
              tunnel: w217 -> [w259]
              tunnel: w215 -> [w258]
              tunnel: w214 -> [w255]
              tunnel: [w253] -> w213 mode=indexing
              tunnel: [w252] -> w212 mode=indexing
              tunnel: [w249] -> w207 mode=indexing
              w265 = dbl[] [] ("Array 4")
              n160 = call-poly <userlib>:"Filter 1D Array__ogtk.vi"("items to filter"=w250, "array"=w258) -> ("filtered item indices"=w257:i32[])  [unwired: 4 in, 1 out]
              n161 = Index Array(array=w257) -> (element=w256:i32)  [unwired: 1 in]
              n162 = Index Array(array=w255, index=w256) -> (element=w251:T6)
              n163 = call "CENTRIOD DETECTION.vi"("Refnum in"=w250, "beam detection para"=w251, "error in (no error)"=w259) -> ("Bounding Rect"=w249:T28, "Particle Reports (Pixels)"=w252:T29, "Centriod"=w276:cluster{"X":dbl, "Y":dbl}, "error out"=w260:errorcluster)  [unwired: 10 in, 3 out]
              n164 = Unbundle By Name(w276) -> ("X"=w273:dbl, "Y"=w272:dbl)
              n165 = Empty Array?(array=w252) -> (empty?=w254:bool)
              n166 = Not Equal To 0?(x=w272) -> (x != 0?=w274:bool)
              n167 = Not Equal To 0?(x=w273) -> (x != 0?=w275:bool)
              n168 = Not(x=w254) -> (.not. x?=w253:bool)
              n169 = And(x=w275, y=w274) -> (x .and. y?=w268:bool)
              n170 = case shown="True" w268 {
                tunnel: w273 -> [_ w309]
                tunnel: w272 -> [_ w308]
                tunnel: w270 -> [w295 w311]
                tunnel: w269 -> [w294 w310]
                tunnel: [w295 w307] -> w267
                tunnel: [w294 w306] -> w264
                tunnel: w249 -> [_ w305]
                tunnel: w262 -> [w293 w298]
                tunnel: [w293 w296] -> w261
                frame False {
                }
                frame True {
                  n171 = Unbundle By Name(w305) -> ("Right"=w304:dbl, "Left"=w303:dbl, "Bottom"=w302:dbl, "Top"=w301:dbl)
                  n172 = Subtract(x=w304, y=w303) -> (x-y=w299:dbl)
                  n173 = Subtract(x=w302, y=w301) -> (x-y=w300:dbl)
                  n174 = Build Array (concatenate)(w311, w309) -> (w307:dbl[])
                  n175 = Multiply(x=w299, y=w300) -> (x*y=w297:dbl)
                  n176 = Build Array (concatenate)(w310, w308) -> (w306:dbl[])
                  n177 = Build Array (concatenate)(w298, w297) -> (w296:dbl[])
                }
              }
              n178 = for {
                tunnel: w267 -> [w286] mode=indexing
                shift-right: [w285] -> w266
                shift-left: w265 -> [w287]
                n179 = Not Equal To 0?(x=w286) -> (x != 0?=w288:bool)
                n180 = case shown="True" w288 {
                  tunnel: w287 -> [w289 w292]
                  tunnel: w286 -> [_ w291]
                  tunnel: [w289 w290] -> w285
                  frame False {
                  }
                  frame True {
                    n181 = Build Array (concatenate)(w292, w291) -> (w290:dbl[])
                  }
                }
              }
              n182 = for {
                tunnel: w264 -> [w278] mode=indexing
                shift-right: [w277] -> w263
                shift-left: w265 -> [w279]
                n183 = Not Equal To 0?(x=w278) -> (x != 0?=w280:bool)
                n184 = case shown="True" w280 {
                  tunnel: w279 -> [w281 w284]
                  tunnel: w278 -> [_ w283]
                  tunnel: [w281 w282] -> w277
                  frame False {
                  }
                  frame True {
                    n185 = Build Array (concatenate)(w284, w283) -> (w282:dbl[])
                  }
                }
              }
              n186 = Array Size(array=w263) -> (size(s)=w271:i32)
            }
            "detected" <- w213
            "Particle Reports (Pixels)" <- w212
            "Box" <- w207
            n187 = Bundle(0, 1, "Centroid X"=w211) -> (→"Waveform Graph":cluster{i32, i32, "Centroid X":dbl[][]})  [unwired: 1 in]
            n188 = call <vilib>:"Clear Errors.vi"("error in (no error)"=w218) -> ("error out"=w216:errorcluster)  [unwired: 6 in]
            n189 = for {
              tunnel: w228 -> [w248] mode=indexing
              tunnel: w227 -> [w247] mode=indexing
              shift-right: [w242] -> w223
              shift-left: "" ("GUIdevice 7") -> [w245]
              tunnel: [w241] -> w225 mode=indexing
              n190 = local read "img to avg"() -> (w240:i32)
              n191 = Greater Or Equal?(x=w248, y=w240) -> (x >= y?=w241:bool)
              n192 = Select(t=w247, s=w241, f="") -> (s? t:f=w243:string)
              n193 = Concatenate Strings(w245, "\t", w243) -> (w242:string)
            }
            n194 = Bundle By Name(cluster=w233, "Centroid X"=w229, "Centroid Y"=w232, "Size"=w219) -> (w231:T30)
            n195 = Or Array Elements(Boolean array=w225) -> (logical OR=w224:bool)
            n196 = case shown="True" w224 {
              tunnel: w223 -> [_ w238]
              tunnel: w222 -> [w234 w236]
              tunnel: [w234 w235] -> w221
              frame False {
              }
              frame True {
                n197 = call <vilib>:"Build State String with Arguments__jki_lib_state_machine.vi"("Arguments (\"\")"=w238, "State"="detected") -> ("State with Arguments"=w237:string)  [unwired: 4 in]
                n198 = call <vilib>:"Add State(s) to Queue__jki_lib_state_machine.vi"("State(s) in (\"\")"=w236, "State(s) at Back (\"\")"=w237) -> ("States Out"=w235:string)  [unwired: 13 in]
              }
            }
          }
          event "stop": Value Change {
            # "Exit Button Value Change (pressed) Event\n(this executes Macro: Exit to terminate the VI)"
            n199 = event-data() -> ()  [unwired: 1 in, 6 out]
            n200 = call <vilib>:"Add State(s) to Queue__jki_lib_state_machine.vi"("State(s) in Front (\"\")"="Macro: Exit", "State(s) in (\"\")"=w316) -> ("States Out"=w315:string)  [unwired: 13 in]
          }
          event "Feedback Global": Value Change {
            # "Exit Button Value Change (pressed) Event\n(this executes Macro: Exit to terminate the VI)"
            n201 = event-data() -> ("NewVal"=w319:bool)  [unwired: 1 in, 5 out]
            n202 = call <vilib>:"Add State(s) to Queue__jki_lib_state_machine.vi"("State(s) in (\"\")"=w322) -> ("States Out"=w321:string)  [unwired: 14 in]
            n203 = Bundle By Name(cluster=w318, "Feedback global"=w319) -> (w317:T30)
          }
          event Value Change {
            n204 = event-data() -> ()  [unwired: 1 in, 6 out]
            n205 = call <vilib>:"Add State(s) to Queue__jki_lib_state_machine.vi"("State(s) in Front (\"\")"="Move Config", "State(s) in (\"\")"=w327) -> ("States Out"=w326:string)  [unwired: 13 in]
          }
          event Value Change {
            n206 = event-data() -> ()  [unwired: 1 in, 6 out]
            n207 = call <vilib>:"Add State(s) to Queue__jki_lib_state_machine.vi"("State(s) in Front (\"\")"="Detection Config", "State(s) in (\"\")"=w332) -> ("States Out"=w331:string)  [unwired: 13 in]
          }
          event "motor config": Value Change {
            n208 = event-data() -> ()  [unwired: 1 in, 6 out]
            n209 = call <vilib>:"Add State(s) to Queue__jki_lib_state_machine.vi"("State(s) in (\"\")"=w337, "State(s) at Back (\"\")"="Motor Config" ("State(s) at Back (\"\")")) -> ("States Out"=w336:string)  [unwired: 13 in]
          }
          event "Reset History": Value Change {
            n210 = event-data() -> ()  [unwired: 1 in, 6 out]
            n211 = call <vilib>:"Add State(s) to Queue__jki_lib_state_machine.vi"("State(s) in (\"\")"=w343, "State(s) at Back (\"\")"="Reset History" ("State(s) at Back (\"\")")) -> ("States Out"=w342:string)  [unwired: 13 in]
            n212 = property on="Reset History" class="Bool (strict)"("Value"=FALSE ("Reset History")) -> ()  [unwired: 2 in, 2 out]
          }
          event "Save Config": Value Change {
            n213 = event-data() -> ()  [unwired: 1 in, 6 out]
            n214 = call <vilib>:"Add State(s) to Queue__jki_lib_state_machine.vi"("State(s) in (\"\")"=w348, "State(s) at Back (\"\")"="Save Config" ("State(s) at Back (\"\")")) -> ("States Out"=w347:string)  [unwired: 13 in]
          }
          event "Load Config": Value Change {
            n215 = event-data() -> ()  [unwired: 1 in, 6 out]
            n216 = call <vilib>:"Add State(s) to Queue__jki_lib_state_machine.vi"("State(s) in (\"\")"=w353, "State(s) at Back (\"\")"="Load Config" ("State(s) at Back (\"\")")) -> ("States Out"=w352:string)  [unwired: 13 in]
          }
          event "active CCDs": Value Change {
            n217 = event-data() -> ("NewVal"=w357:i32)  [unwired: 1 in, 5 out]
            n218 = Index Array(array=w358, index=w357) -> (element=w355:string)
            n219 = call <vilib>:"Build State String with Arguments__jki_lib_state_machine.vi"("Arguments (\"\")"=w355, "State"="active" ("State(s) at Back (\"\")")) -> ("State with Arguments"=w354:string)  [unwired: 4 in]
            n220 = call <vilib>:"Add State(s) to Queue__jki_lib_state_machine.vi"("State(s) in (\"\")"=w362, "State(s) at Back (\"\")"=w354) -> ("States Out"=w361:string)  [unwired: 13 in]
          }
          event Panel Close? {
            # "Discard the event because we'll close the front panel ourselves in Macro: Exit"
            # "Close Panel button (pressed) Event\n(this executes Macro: Exit to terminate the VI)"
            n221 = event-data() -> ()  [unwired: 1 in, 1 out]
            n222 = call <vilib>:"Add State(s) to Queue__jki_lib_state_machine.vi"("State(s) in Front (\"\")"="Macro: Exit", "State(s) in (\"\")"=w368) -> ("States Out"=w367:string)  [unwired: 13 in]
            n223 = event-data("Discard?"=TRUE) -> ()  [unwired: 1 in, 1 out]
          }
        }
      }
      frame "---------- Core ----------" {
        # "Do not put any code in this frame.\n(it is a separator no-op)"
        n224 = call <vilib>:"Add State(s) to Queue__jki_lib_state_machine.vi"("State(s) in (\"\")"=w372) -> ("States Out"=w371:string)  [unwired: 14 in]
      }
      frame Default {
        w382 = 42 items=["No error", "Argument error", "Memory is full", "Out of zone", "End of file", "File already open", "Generic file I/O error", "File not found", "File permission error", "Disk is full", "Duplicate path", "Too many files open", "System feature not enabled", "Resource file not found", "Cannot add resource", "Resource not found", "Image not found", "Image memory error", "Pen does not exist", "Config type invalid", "Config token not found", "Config parse error", "Config memory error", "Bad external code format", "Bad external code offset", "External code not present", "Null window", "Destroy window error", "Null menu", "Print aborted", "Bad print record", "Print driver error", "Windows error during printing", "Memory error during printing", "Print dialog error", "Generic print error", "Invalid device refnum", "Device not found", "Device parameter error", "Device unit error", "Cannot open device", "Device call aborted", "Generic error", "Cancelled by user", "Object ID too low", "Object ID too high", "Object not in heap", "Unknown heap", "Unknown object (invalid DefProc)", "Unknown object (DefProc not in table)", "Message out of range", "Invalid (null) method", "Unknown message", "Manager call not supported", "Bad address", "Network operation in progress", "Network operation timed out", "Connection is busy", "Network attribute not supported", "Network error", "Address in use", "System out of memory", "Connection aborted", "Connection refused", "Not connected", "Already connected", "Connection closed", "Initialization error (interapplication manager)", "Bad occurrence", "Wait on unbound occurrence handler", "Occurrence queue overflow", "Datalog type conflict", "Unused", "Unrecognized type (interapplication manager)", "Memory corrupt", "Failed to make temporary DLL", "Old CIN version", "Drag socket not found", "Failed to load drop-object", "Failed to register OLE object", "Failed to release OLE object", "Format specifier type mismatch", "Unknown format specifier", "Too few format specifiers", "Too many format specifiers", "Scan failed", "Newer CIN version", "Error converting to variant", "Runtime menu error", "Password tampered", "Variant attribute not found", "Incompatible variant data type", "Event data is not available", "Event Store is not present", "Occurrence is not found", "Event Queue is not created", "Event info is not available", "Refnum passed is NULL", "Error retrieving Class GUID", "Error retrieving CoClass GUID", "Error retrieving TypeLib GUID.", "Bad built application magic bytes.", "Specific driver is different from the specific driver associated with the Logical Name.", "There is no session opened to the class driver.", "Max Error", "MAX - Error with config objects", "MAX - Error loading configuration", "MAX - Group not supported"]
        # "Current State"
        # "Do not delete, rename, or modify this frame.\n(this is used to capture unhandled states and typos)"
        # "Handle mistyped state name (developer tool)"
        n225 = Format Into String(format string="Software Exception: Unhandled State \"%s\"." ("message"), error in=w378, w373) -> (resulting string=w381:string, error out=w380:errorcluster)  [unwired: 1 in]
        n226 = call <vilib>:"Error Cluster From Error Code.vi"("show call chain? (False)"=TRUE, "error in (no error)"=w380, "error message (\"\")"=w381, "error code (0)"=w382) -> ("error out"=w379:errorcluster)  [unwired: 5 in]
        n227 = call <vilib>:"Add State(s) to Queue__jki_lib_state_machine.vi"("State(s) in (\"\")"=w377) -> ("States Out"=w376:string)  [unwired: 14 in]
      }
      frame "Initialize Core Data" {
        # "Do not delete, rename, or modify this frame.\n(this is used to determine panel behavior on exit)"
        # "originally closed?"
        # "exe?"
        # "If panel starts closed or is an EXE, then close it when we exit"
        n228 = property class="VI"() -> ("Front Panel.Open"=w392:bool)  [unwired: 2 in, 2 out]
        n229 = property class="App"() -> ("App.Kind"=w391:T25)  [unwired: 2 in, 2 out]
        n230 = control-ref of="Current VI Reference"() -> (w386:refnum<vi>)
        n231 = Not(x=w392) -> (.not. x?=w389:bool)
        n232 = Equal?(x=w391, y=T25."Run Time System" ("Application:Kind")) -> (x = y?=w388:bool)
        n233 = Or(x=w389, y=w388) -> (x .or. y?=w387:bool)
        n234 = Bundle By Name(cluster=w385, "Core.Current VI Reference"=w386, "Core.Close Panel on Exit?"=w387) -> (w384:T30)
        n235 = call <vilib>:"Add State(s) to Queue__jki_lib_state_machine.vi"("State(s) in (\"\")"=w395) -> ("States Out"=w394:string)  [unwired: 14 in]
      }
      frame "Error Handler" {
        # "Unhandled Error -- Display it"
        # "Handle any errors here.\nYou can also output any states to clean-up after errors occur"
        # "Clear error"
        n236 = call <vilib>:"General Error Handler.vi"("error in (no error)"=w397) -> ()  [unwired: 10 in, 5 out]
        n237 = call <vilib>:"Add State(s) to Queue__jki_lib_state_machine.vi"("State(s) in Front (\"\")"="/* Post Error States", "State(s) in (\"\")"=w401) -> ("States Out"=w400:string)  [unwired: 13 in]
      }
      frame "Exit" {
        # "Do not put any code in this frame.\n(No errors that occur here will be handled.)"
        n238 = call <vilib>:"Add State(s) to Queue__jki_lib_state_machine.vi"("State(s) in (\"\")"=w406) -> ("States Out"=w405:string)  [unwired: 14 in]
      }
      frame "---------- Data ----------" {
        # "Do not put any code in this frame.\n(It is a separator no-op. You can make a copy of this frame to create a new Data frame)"
        n239 = call <vilib>:"Add State(s) to Queue__jki_lib_state_machine.vi"("State(s) in (\"\")"=w410) -> ("States Out"=w409:string)  [unwired: 14 in]
      }
      frame "Data: Initialize" {
        w414 = FALSE  # Feedback global
        w416 = 0  # active ccd
        w428 = 20  # img to avg
        w429 = T31 {"Current VI Reference"=refnum, "Close Panel on Exit?"=FALSE}  # Core
        # "Initialize the shift-register data, here.\n(data names are defined by what you wire into the bundle function)"
        n240 = Bundle("Core"=w429, "detection para"="detection para", "Centroid X"="Centroid X", "Centroid Y"="Centroid Y", "img to avg"=w428, "Mean Centroid X"="Mean Centroid X", "Mean Centroid Y"="Mean Centroid Y", "Offset X"="Offset X", "Offset Y"="Offset Y", "Offset X stats"="Offset X stats", "Offset Y stats"="Offset Y stats", "Size"="Size", "Mean Size"="Mean Size", "Time"="Time", "move properties"="move properties", "active axis refs 2"="active axis refs 2", "active ccd"=w416, "Feedback global"=w414) -> (w425:T30)  [unwired: 1 in]
        n241 = call <vilib>:"Add State(s) to Queue__jki_lib_state_machine.vi"("State(s) in (\"\")"=w432) -> ("States Out"=w431:string)  [unwired: 14 in]
      }
      frame "Data: Cleanup" {
        # "Cleanup any data and references, here.\n(this is called automatically, by the Macro: Exit)"
        n242 = Unbundle By Name(w433) -> ("Core.Current VI Reference"=w434:refnum<vi>)
        n243 = Close Reference(reference=w434, error in (no error)=w436) -> (error out=w435:errorcluster)
        n244 = call <vilib>:"Add State(s) to Queue__jki_lib_state_machine.vi"("State(s) in (\"\")"=w438) -> ("States Out"=w437:string)  [unwired: 14 in]
      }
      frame "---------- UI ----------" {
        # "Do not put any code in this frame.\n(It is a separator no-op. You can make a copy of this frame to create a new UI frame)"
        n245 = call <vilib>:"Add State(s) to Queue__jki_lib_state_machine.vi"("State(s) in (\"\")"=w442) -> ("States Out"=w441:string)  [unwired: 14 in]
      }
      frame "UI: Initialize" {
        # "Initialize the User Interface, here.\n(this is called automatically, by the Macro: Init)"
        n246 = call <vilib>:"Add State(s) to Queue__jki_lib_state_machine.vi"("State(s) in (\"\")"=w446) -> ("States Out"=w445:string)  [unwired: 14 in]
      }
      frame "UI: Cursor Set" {
        # "Argument"
        # "Set and Unset Cursor Busy.\n(Usage: \"UI: Cursor Set >> Busy|Idle\")"
        n247 = case shown="\"Idle\", Default" w447 {
          tunnel: w449 -> [w454 w456]
          tunnel: [w453 w455] -> w448
          frame "Idle", Default {
            n248 = call <vilib>:"Unset Busy.vi"("error in (no error)"=w454) -> ("error out"=w453:errorcluster)  [unwired: 10 in]
          }
          frame "Busy" {
            n249 = call <vilib>:"Set Busy.vi"("error in (no error)"=w456) -> ("error out"=w455:errorcluster)  [unwired: 9 in, 1 out]
          }
        }
        n250 = call <vilib>:"Add State(s) to Queue__jki_lib_state_machine.vi"("State(s) in (\"\")"=w452) -> ("States Out"=w451:string)  [unwired: 14 in]
      }
      frame "UI: Front Panel State" {
        # "Argument"
        # "Set Front Panel Open or Closed\n(Usage: \"UI: Front Panel State >> Open|Close\")"
        n251 = Unbundle By Name(w457) -> ("Core.Current VI Reference"=w459:refnum<vi>)
        n252 = case shown="\"Open\", Default" w458 {
          tunnel: w461 -> [w467 w478]
          tunnel: [w468 w479] -> w460
          tunnel: w459 -> [_ _]
          frame "Open", Default {
            n253 = property class="VI"(error in=w467) -> (reference out=w465:refnum<vi>, error out=w466:errorcluster, "Front Panel.Open"=w464:bool)  [unwired: 1 in]
            n254 = case shown="False" w464 {
              tunnel: [w471 w474] -> w468
              tunnel: w466 -> [w470 w474]
              tunnel: w465 -> [w469 _]
              frame False {
                n255 = invoke class="VI" method="FP.Open"(reference=w469, error in=w470, "Activate"=TRUE, "State"=T26."Standard") -> (error out=w471:errorcluster)  [unwired: 1 in, 4 out]
              }
              frame True {
              }
            }
          }
          frame "Close" {
            n256 = property class="VI"(error in=w478) -> (reference out=w476:refnum<vi>, error out=w477:errorcluster, "Front Panel.Open"=w475:bool)  [unwired: 1 in]
            n257 = case shown="True" w475 {
              tunnel: [w480 w483] -> w479
              tunnel: w477 -> [w480 w482]
              tunnel: w476 -> [_ w481]
              frame False {
              }
              frame True {
                n258 = invoke class="VI" method="FP.Close"(reference=w481, error in=w482) -> (error out=w483:errorcluster)  [unwired: 1 in, 2 out]
              }
            }
          }
        }
        n259 = call <vilib>:"Add State(s) to Queue__jki_lib_state_machine.vi"("State(s) in (\"\")"=w463) -> ("States Out"=w462:string)  [unwired: 14 in]
      }
      frame "---------- Macro ----------" {
        # "Do not put any code in this frame.\n(It is a separator no-op. You can make a copy of this frame to create a new Macro frame)"
        n260 = call <vilib>:"Add State(s) to Queue__jki_lib_state_machine.vi"("State(s) in (\"\")"=w487) -> ("States Out"=w486:string)  [unwired: 14 in]
      }
      frame "Macro: Initialize" {
        w488 = "Data: Initialize\nInitialize Core Data\nUI: Initialize\nUI: Front Panel State >> Open\nMotor Config\nMove Config\nDetection Config"  # Data: Initialize Initialize Core Data UI: Initialize UI: Front Panel State >> Open Motor Config Move Config Detection Config
        # "Initialization Macro\n(This is called once, when the VI starts)"
        n261 = call <vilib>:"Add State(s) to Queue__jki_lib_state_machine.vi"("State(s) in Front (\"\")"=w488, "State(s) in (\"\")"=w492) -> ("States Out"=w491:string)  [unwired: 13 in]
      }
      frame "Macro: Exit" {
        # "Exit Macro\n(This is called once, when the VI exits)"
        n262 = Unbundle By Name(w494) -> ("Core.Close Panel on Exit?"=w493:bool)
        n263 = Select(t="UI: Front Panel State >> Close", s=w493, f="") -> (s? t:f=w497:string)
        n264 = call <vilib>:"Add State(s) to Queue__jki_lib_state_machine.vi"("State(s) in (\"\")"=w497, "State(s) at Back (\"\")"="Data: Cleanup\nExit") -> ("States Out"=w495:string)  [unwired: 13 in]
        n265 = call <vilib>:"Add State(s) to Queue__jki_lib_state_machine.vi"("State(s) in Front (\"\")"=w495, "State(s) in (\"\")"=w502) -> ("States Out"=w501:string)  [unwired: 13 in]
      }
      frame "---------- New Category ----------" {
        # "Template Separator\n(You can make a copy of, or modify, this frame)"
        n266 = call <vilib>:"Add State(s) to Queue__jki_lib_state_machine.vi"("State(s) in (\"\")"=w506) -> ("States Out"=w505:string)  [unwired: 14 in]
      }
      frame "detected" {
        # "Your code here.\n(You can make a copy of, or modify, this frame)"
        n267 = Spreadsheet String To Array(format string="%s", spreadsheet string=w550, array type (2D Dbl)=string[] []) -> (array=w548:string[])  [unwired: 1 in]
        "array" <- w548
        n268 = for {
          tunnel: w548 -> [w633] mode=indexing
          tunnel: w547 -> [w632]
          tunnel: [w631] -> w539 mode=indexing
          n269 = Equal?(x=w633, y=w632) -> (x = y?=w631:bool[])
        }
        n270 = Unbundle By Name(w536) -> ("Offset X"=w535:dbl[][], "Offset Y"=w534:dbl[][], "Size"=w533:dbl[][], "Mean Size"=w532:dbl[][], "Time"=w528:timestamp[][])
        n271 = Unbundle By Name(w536) -> ("Mean Centroid X"=w544:dbl[][], "Mean Centroid Y"=w543:dbl[][], "Centroid X"=w546:dbl[][], "Centroid Y"=w545:dbl[][])
        n272 = Transpose 2D Array(2D array=w539) -> (transposed array=w538:bool[][])
        n273 = for {
          tunnel: w546 -> [w579]
          tunnel: w545 -> [w578]
          tunnel: w544 -> [w577]
          tunnel: w543 -> [w576]
          tunnel: [w575] -> w541 mode=indexing
          tunnel: [w574] -> w540 mode=indexing
          tunnel: w538 -> [w571] mode=indexing
          tunnel: w537 -> [w570] mode=indexing
          tunnel: w535 -> [w569]
          tunnel: w534 -> [w568]
          tunnel: [w567] -> w527 mode=indexing
          tunnel: [w566] -> w525 mode=indexing
          tunnel: w533 -> [w565]
          tunnel: w532 -> [w564]
          tunnel: [w563] -> w531 mode=indexing
          tunnel: w528 -> [w562]
          tunnel: [w561] -> w526 mode=indexing
          i -> [w572]
          n274 = Or Array Elements(Boolean array=w571) -> (logical OR=w573:bool)
          n275 = case shown="True" w573 {
            tunnel: w579 -> [_ w630]
            tunnel: w578 -> [_ w629]
            tunnel: w577 -> [w594 w626]
            tunnel: w576 -> [w593 w625]
            tunnel: [w592 w622] -> w575
            tunnel: [w591 w621] -> w574
            tunnel: w572 -> [w583 w602]
            tunnel: w570 -> [_ w620]
            tunnel: w569 -> [w590 w617]
            tunnel: w568 -> [w589 w616]
            tunnel: [w588 w611] -> w567
            tunnel: [w587 w610] -> w566
            tunnel: w565 -> [_ w609]
            tunnel: w564 -> [w586 w607]
            tunnel: [w585 w604] -> w563
            tunnel: w562 -> [w584 w601]
            tunnel: [w580 w599] -> w561
            frame False {
              n276 = Index Array(array=w584, index (row)=w583) -> (element=w581:timestamp[])  [unwired: 1 in]
              n277 = Index Array(array=w594, index (row)=w583) -> (element=w592:dbl[])  [unwired: 1 in]
              n278 = Index Array(array=w593, index (row)=w583) -> (element=w591:dbl[])  [unwired: 1 in]
              n279 = Index Array(array=w590, index (row)=w583) -> (element=w588:dbl[])  [unwired: 1 in]
              n280 = Index Array(array=w586, index (row)=w583) -> (element=w585:dbl[])  [unwired: 1 in]
              n281 = Index Array(array=w589, index (row)=w583) -> (element=w587:dbl[])  [unwired: 1 in]
              n282 = Get Date/Time In Seconds() -> (seconds since 1Jan1904=w582:timestamp)
              n283 = Build Array (concatenate)(w581, w582) -> (w580:timestamp[])
            }
            frame True {
              n284 = Unbundle By Name(w620) -> ("Target.X::8"=w598:refnum<vi>, "Target.Y::8"=w597:refnum<vi>)
              n285 = Index Array(array=w626, index (row)=w602) -> (element=w623:dbl[])  [unwired: 1 in]
              n286 = Index Array(array=w625, index (row)=w602) -> (element=w624:dbl[])  [unwired: 1 in]
              n287 = Index Array(array=w630, index (row)=w602) -> (element=w628:dbl[])  [unwired: 1 in]
              n288 = Index Array(array=w629, index (row)=w602) -> (element=w627:dbl[])  [unwired: 1 in]
              n289 = Index Array(array=w617, index (row)=w602) -> (element=w614:dbl[])  [unwired: 1 in]
              n290 = Index Array(array=w616, index (row)=w602) -> (element=w613:dbl[])  [unwired: 1 in]
              n291 = Index Array(array=w609, index (row)=w602) -> (element=w608:dbl[])  [unwired: 1 in]
              n292 = Index Array(array=w607, index (row)=w602) -> (element=w606:dbl[])  [unwired: 1 in]
              n293 = Index Array(array=w601, index (row)=w602) -> (element=w600:timestamp[])  [unwired: 1 in]
              n294 = property class="DigNum (strict)"(reference=w598) -> ("Value"=w596:dbl)  [unwired: 1 in, 2 out]
              n295 = property class="DigNum (strict)"(reference=w597) -> ("Value"=w595:dbl)  [unwired: 1 in, 2 out]
              n296 = call <vilib>:"Std Deviation and Variance.vi"("X"=w628) -> ("mean"=w619:dbl)  [unwired: 1 in, 2 out]
              n297 = call <vilib>:"Std Deviation and Variance.vi"("X"=w627) -> ("mean"=w618:dbl)  [unwired: 1 in, 2 out]
              n298 = call <vilib>:"Std Deviation and Variance.vi"("X"=w608) -> ("mean"=w605:dbl)  [unwired: 1 in, 2 out]
              n299 = Get Date/Time In Seconds() -> (seconds since 1Jan1904=w603:timestamp)
              n300 = Subtract(x=w596, y=w619) -> (x-y=w615:dbl)
              n301 = Subtract(x=w595, y=w618) -> (x-y=w612:dbl)
              n302 = Build Array (concatenate)(w623, w619) -> (w622:dbl[])
              n303 = Build Array (concatenate)(w624, w618) -> (w621:dbl[])
              n304 = Build Array (concatenate)(w606, w605) -> (w604:dbl[])
              n305 = Build Array (concatenate)(w600, w603) -> (w599:timestamp[])
              n306 = Build Array (concatenate)(w614, w615) -> (w611:dbl[])
              n307 = Build Array (concatenate)(w613, w612) -> (w610:dbl[])
            }
          }
        }
        n308 = call <vilib>:"Add State(s) to Queue__jki_lib_state_machine.vi"("State(s) in (\"\")"=w554, "State(s) at Back (\"\")"="Check Move" ("State(s) at Back (\"\")")) -> ("States Out"=w553:string)  [unwired: 13 in]
        n309 = local read "Centroid X"() -> (w524:dbl[][])
        n310 = local read "Size"() -> (w530:dbl[][])
        n311 = for {
          tunnel: w527 -> [w560] mode=indexing
          tunnel: w526 -> [w558] mode=indexing
          tunnel: w525 -> [w559] mode=indexing
          tunnel: [w555] -> w523 mode=indexing
          n312 = Bundle(w558, "Offset Y"=w559) -> (w556:cluster{timestamp[], "Offset Y":dbl[]})  [unwired: 1 in]
          n313 = Bundle(w558, "Offset X"=w560) -> (w557:cluster{timestamp[], "Offset X":dbl[]})  [unwired: 1 in]
          n314 = Build Array(w557, w556) -> (w555:cluster{timestamp[], "Offset Y":dbl[]}[])
        }
        n315 = Bundle By Name(cluster=w536, "Centroid X"=w524, "Centroid Y"=w524, "Mean Centroid X"=w541, "Mean Centroid Y"=w540, "Offset X"=w527, "Offset Y"=w525, "Mean Size"=w531, "Size"=w530, "Time"=w526) -> (w542:T30)
        n316 = Index Array(array=w523, index (row) #1=0 ("index (row)"), index (row) #2=1 ("index (row)"), index (row) #3=2 ("index (row)"), index (row) #4=3 ("index (row)"), index (row) #5=4 ("index (row)"), index (row) #6=5 ("index (row)"), index (row) #7=6 ("index (row)"), index (row) #8=7 ("index (row)")) -> (element #1=→"CCD 1":cluster{timestamp[], "Offset Y":dbl[]}[], element #2=→"CCD 2":cluster{timestamp[], "Offset Y":dbl[]}[], element #3=→"CCD 3":cluster{timestamp[], "Offset Y":dbl[]}[], element #4=→"CCD 4":cluster{timestamp[], "Offset Y":dbl[]}[], element #5=→"CCD 5":cluster{timestamp[], "Offset Y":dbl[]}[], element #6=→"CCD 6":cluster{timestamp[], "Offset Y":dbl[]}[], element #7=→"CCD 7":cluster{timestamp[], "Offset Y":dbl[]}[], element #8=→"CCD 8":cluster{timestamp[], "Offset Y":dbl[]}[])  [unwired: 8 in]
      }
      frame "Check Move" {
        # "Your code here.\n(You can make a copy of, or modify, this frame)"
        n317 = Unbundle By Name(w647) -> ("Mean Size"=w657:dbl[][], "move properties"=w660:T1[], "Offset X"=w659:dbl[][], "Offset Y"=w658:dbl[][])
        n318 = for {
          tunnel: w660 -> [w712] mode=indexing
          tunnel: w659 -> [w716] mode=indexing
          tunnel: w658 -> [w715] mode=indexing
          tunnel: w657 -> [w705] mode=indexing
          tunnel: [w697] -> w656 mode=indexing
          tunnel: [w690] -> w655 mode=indexing
          tunnel: w654 -> [w687] mode=indexing
          tunnel: [w694] -> w653 mode=indexing
          tunnel: [w689] -> w650 mode=indexing
          n319 = Unbundle By Name(w712) -> ("Tolerance [%]"=w708:dbl)
          n320 = Reverse 1D Array(array=w716) -> (reversed array=w714:dbl[])
          n321 = Reverse 1D Array(array=w715) -> (reversed array=w713:dbl[])
          n322 = Reverse 1D Array(array=w705) -> (reversed array=w707:dbl[])
          n323 = Index Array(array=w714) -> (element=w711:dbl)  [unwired: 1 in]
          n324 = Index Array(array=w713) -> (element=w710:dbl)  [unwired: 1 in]
          n325 = Index Array(array=w707) -> (element=w706:dbl)  [unwired: 1 in]
          n326 = Absolute Value(x=w711) -> (abs(x)=w695:dbl)
          n327 = Absolute Value(x=w710) -> (abs(x)=w688:dbl)
          n328 = Square Root(x=w706) -> (sqrt(x)=w704:dbl)
          n329 = Divide(x=w708, y=100.0) -> (x/y=w703:dbl)
          n330 = Multiply(x=w704, y=w703) -> (x*y=w702:dbl)
          n331 = Not Equal To 0?(x=w688) -> (x != 0?=w701:bool)
          n332 = Not Equal To 0?(x=w695) -> (x != 0?=w700:bool)
          n333 = Greater Or Equal?(x=w695, y=w702) -> (x >= y?=w699:bool)
          n334 = Greater Or Equal?(x=w688, y=w702) -> (x >= y?=w698:bool)
          n335 = And(x=w700, y=w699) -> (x .and. y?=w697:bool)
          n336 = And(x=w698, y=w701) -> (x .and. y?=w690:bool)
          n337 = Boolean To (0,1)(Boolean=w697) -> (0, 1=w696:i16)
          n338 = Boolean To (0,1)(Boolean=w690) -> (0, 1=w691:i16)
          n339 = Multiply(x=w696, y=w695) -> (x*y=w693:dbl)
          n340 = Multiply(x=w691, y=w688) -> (x*y=w692:dbl)
          n341 = Bundle(w693, "GUIdevice 8"=w687) -> (w694:cluster{dbl, "GUIdevice 8":string})  [unwired: 1 in]
          n342 = Bundle(w692, "GUIdevice 8"=w687) -> (w689:cluster{dbl, "GUIdevice 8":string})  [unwired: 1 in]
        }
        "required X" <- w656
        "required Y" <- w655
        n343 = Sort 1D Array(array=w650) -> (sorted array=w651:cluster{dbl, "GUIdevice 8":string}[])
        n344 = Sort 1D Array(array=w653) -> (sorted array=w652:cluster{dbl, "GUIdevice 8":string}[])
        n345 = Reverse 1D Array(array=w651) -> (reversed array=w637:cluster{dbl, "GUIdevice 8":string}[])
        "sorted array Y" <- w637
        n346 = Reverse 1D Array(array=w652) -> (reversed array=w645:cluster{dbl, "GUIdevice 8":string}[])
        "sorted array X" <- w645
        n347 = Empty Array?(array=w645) -> (empty?=w641:bool)
        n348 = Empty Array?(array=w637) -> (empty?=w635:bool)
        n349 = Index Array(array=w645) -> (element=w644:cluster{dbl, "GUIdevice 8":string})  [unwired: 1 in]
        n350 = Index Array(array=w637) -> (element=w638:cluster{dbl, "GUIdevice 8":string})  [unwired: 1 in]
        n351 = Unbundle(w644) -> (w643:dbl)  [unwired: 1 out]
        n352 = Unbundle(w638) -> (w639:dbl)  [unwired: 1 out]
        n353 = Unbundle By Name(w647) -> ("Feedback global"=w646:bool)
        n354 = Equal To 0?(x=w643) -> (x = 0?=w642:bool)
        n355 = Equal To 0?(x=w639) -> (x = 0?=w636:bool)
        n356 = Or(x=w642, y=w641) -> (x .or. y?=w640:bool)
        n357 = Or(x=w636, y=w635) -> (x .or. y?=w634:bool)
        n358 = case shown="True" w646 {
          tunnel: w640 -> [_ w670]
          tunnel: w645 -> [_ w669]
          tunnel: w634 -> [_ w667]
          tunnel: w637 -> [_ w666]
          tunnel: w649 -> [w663 w665]
          tunnel: [w663 w664] -> w648
          frame False {
          }
          frame True {
            n359 = case shown="False" w670 {
              tunnel: w669 -> [w685 _]
              tunnel: w665 -> [w681 w686]
              tunnel: [w679 w686] -> w668
              frame False {
                n360 = Index Array(array=w685) -> (element=w684:cluster{dbl, "GUIdevice 8":string})  [unwired: 1 in]
                n361 = Unbundle By Name(w684) -> ("GUIdevice 8"=w683:string)
                n362 = call <vilib>:"Build State String with Arguments__jki_lib_state_machine.vi"("Arguments (\"\")"=w683, "State"="Move X") -> ("State with Arguments"=w680:string)  [unwired: 4 in]
                n363 = call <vilib>:"Add State(s) to Queue__jki_lib_state_machine.vi"("State(s) in (\"\")"=w681, "State(s) at Back (\"\")"=w680) -> ("States Out"=w679:string)  [unwired: 13 in]
              }
              frame True {
              }
            }
            n364 = case shown="False" w667 {
              tunnel: w666 -> [w677 _]
              tunnel: w668 -> [w673 w678]
              tunnel: [w671 w678] -> w664
              frame False {
                n365 = Index Array(array=w677) -> (element=w676:cluster{dbl, "GUIdevice 8":string})  [unwired: 1 in]
                n366 = Unbundle By Name(w676) -> ("GUIdevice 8"=w675:string)
                n367 = call <vilib>:"Build State String with Arguments__jki_lib_state_machine.vi"("Arguments (\"\")"=w675, "State"="Move Y") -> ("State with Arguments"=w672:string)  [unwired: 4 in]
                n368 = call <vilib>:"Add State(s) to Queue__jki_lib_state_machine.vi"("State(s) in (\"\")"=w673, "State(s) at Back (\"\")"=w672) -> ("States Out"=w671:string)  [unwired: 13 in]
              }
              frame True {
              }
            }
          }
        }
        n369 = call <vilib>:"Add State(s) to Queue__jki_lib_state_machine.vi"("State(s) in (\"\")"=w649, "State(s) at Back (\"\")"=w648) -> ("States Out"=w662:string)  [unwired: 13 in]
      }
      frame "Move X" {
        # "Your code here.\n(You can make a copy of, or modify, this frame)"
        n370 = Unbundle By Name(w734) -> ("Offset X"=w733:dbl[][])
        n371 = call-poly <userlib>:"Filter 1D Array__ogtk.vi"("items to filter"=w735, "array"=w739) -> ("filtered item indices"=w721:i32[])  [unwired: 4 in, 1 out]
        n372 = Unbundle By Name(w734) -> ("active axis refs 2"=w738:T11, "move properties"=w720:T1[])
        "move properties 2" <- w720
        n373 = for {
          tunnel: w721 -> [w744] mode=indexing
          tunnel: w720 -> [w748]
          shift-right: [w743] -> w718
          shift-left: i32[] [] ("filtered item indices") -> [w746]
          n374 = Index Array(array=w748, index=w744) -> (element=w747:T1)
          n375 = Unbundle By Name(w747) -> ("enable feedback"=w745:bool)
          n376 = case shown="True" w745 {
            tunnel: w746 -> [w749 w752]
            tunnel: w744 -> [_ w751]
            tunnel: [w749 w750] -> w743
            frame False {
            }
            frame True {
              n377 = Build Array (concatenate)(w752, w751) -> (w750:i32[])
            }
          }
        }
        n378 = Index Array(array=w718) -> (element=w717:i32)  [unwired: 1 in]
        n379 = Index Array(array=w733, index (row)=w717) -> (element=w732:dbl[])  [unwired: 1 in]
        n380 = Reverse 1D Array(array=w732) -> (reversed array=w731:dbl[])
        n381 = Index Array(array=w738, index=w717) -> (element=w737:cluster{"Ref X":refnum<vi>, "Ref Y":refnum<vi>})
        n382 = Index Array(array=w731) -> (element=w729:dbl)  [unwired: 1 in]
        n383 = Index Array(array=w720, index=w717) -> (element=w736:T1)
        n384 = Unbundle By Name(w737) -> ("Ref X"=w725:refnum<vi>, "Ref Y"=w724:refnum<vi>)
        n385 = Unbundle By Name(w736) -> ("Invert Direction X"=w726:bool, "Invert Axis"=w730:bool, "Stepsize"=w727:dbl, "enable feedback"=w723:bool)
        n386 = Greater Or Equal To 0?(x=w729) -> (x >= 0?=w728:bool)
        n387 = call <vilib>:"Add State(s) to Queue__jki_lib_state_machine.vi"("State(s) in Front (\"\")"="Wait" ("State(s) in Front (\"\")"), "State(s) in (\"\")"=w742) -> ("States Out"=w741:string)  [unwired: 13 in]
        n388 = case shown="True" w723 {
          tunnel: w730 -> [_ w758]
          tunnel: w728 -> [_ w757]
          tunnel: w727 -> [_ w756]
          tunnel: w726 -> [_ w755]
          tunnel: w725 -> [_ w754]
          tunnel: w724 -> [_ w753]
          frame False {
          }
          frame True {
            n389 = case shown="False" w757 {
              tunnel: w755 -> [w766 w788]
              tunnel: w756 -> [w764 w786]
              tunnel: w758 -> [w763 w785]
              tunnel: w758 -> [w762 w784]
              tunnel: w754 -> [w760 w782]
              tunnel: w753 -> [w759 w781]
              frame True {
                n390 = case shown="False" w763 {
                  tunnel: [w777 w779] -> w765
                  tunnel: w760 -> [w778 _]
                  tunnel: w759 -> [_ w780]
                  frame False {
                    n391 = property class="DigNum (strict)"(reference=w778) -> ("Value"=w777:dbl)  [unwired: 1 in, 2 out]
                  }
                  frame True {
                    n392 = property class="DigNum (strict)"(reference=w780) -> ("Value"=w779:dbl)  [unwired: 1 in, 2 out]
                  }
                }
                n393 = case shown="False" w766 {
                  tunnel: w765 -> [w773 w776]
                  tunnel: w764 -> [w772 w775]
                  tunnel: [w771 w774] -> w761
                  frame False {
                    n394 = Add(x=w773, y=w772) -> (x+y=w771:dbl)
                  }
                  frame True {
                    n395 = Subtract(x=w776, y=w775) -> (x-y=w774:dbl)
                  }
                }
                n396 = case shown="False" w762 {
                  tunnel: w761 -> [w767 w769]
                  tunnel: w760 -> [w768 _]
                  tunnel: w759 -> [_ w770]
                  frame False {
                    n397 = property class="DigNum (strict)"(reference=w768, "Val(Sgnl)"=w767) -> ()  [unwired: 1 in, 2 out]
                  }
                  frame True {
                    n398 = property class="DigNum (strict)"(reference=w770, "Val(Sgnl)"=w769) -> ()  [unwired: 1 in, 2 out]
                  }
                }
              }
              frame False {
                n399 = case shown="False" w785 {
                  tunnel: [w799 w801] -> w787
                  tunnel: w782 -> [w800 _]
                  tunnel: w781 -> [_ w802]
                  frame False {
                    n400 = property class="DigNum (strict)"(reference=w800) -> ("Value"=w799:dbl)  [unwired: 1 in, 2 out]
                  }
                  frame True {
                    n401 = property class="DigNum (strict)"(reference=w802) -> ("Value"=w801:dbl)  [unwired: 1 in, 2 out]
                  }
                }
                n402 = case shown="False" w788 {
                  tunnel: w787 -> [w795 w798]
                  tunnel: w786 -> [w794 w797]
                  tunnel: [w793 w796] -> w783
                  frame False {
                    n403 = Subtract(x=w795, y=w794) -> (x-y=w793:dbl)
                  }
                  frame True {
                    n404 = Add(x=w798, y=w797) -> (x+y=w796:dbl)
                  }
                }
                n405 = case shown="False" w784 {
                  tunnel: w783 -> [w789 w791]
                  tunnel: w782 -> [w790 _]
                  tunnel: w781 -> [_ w792]
                  frame False {
                    n406 = property class="DigNum (strict)"(reference=w790, "Val(Sgnl)"=w789) -> ()  [unwired: 1 in, 2 out]
                  }
                  frame True {
                    n407 = property class="DigNum (strict)"(reference=w792, "Val(Sgnl)"=w791) -> ()  [unwired: 1 in, 2 out]
                  }
                }
              }
            }
          }
        }
        "Arguments X" <- w735
      }
      frame "Move Y" {
        # "Your code here.\n(You can make a copy of, or modify, this frame)"
        n408 = Unbundle By Name(w820) -> ("Offset Y"=w819:dbl[][])
        n409 = call-poly <userlib>:"Filter 1D Array__ogtk.vi"("items to filter"=w821, "array"=w825) -> ("filtered item indices"=w808:i32[])  [unwired: 4 in, 1 out]
        n410 = Unbundle By Name(w820) -> ("active axis refs 2"=w824:T11, "move properties"=w806:T1[])
        n411 = for {
          tunnel: w808 -> [w830] mode=indexing
          tunnel: w806 -> [w834]
          shift-right: [w829] -> w807
          shift-left: i32[] [] ("filtered item indices") -> [w832]
          n412 = Index Array(array=w834, index=w830) -> (element=w833:T1)
          n413 = Unbundle By Name(w833) -> ("enable feedback"=w831:bool)
          n414 = case shown="True" w831 {
            tunnel: w832 -> [w835 w838]
            tunnel: w830 -> [_ w837]
            tunnel: [w835 w836] -> w829
            frame False {
            }
            frame True {
              n415 = Build Array (concatenate)(w838, w837) -> (w836:i32[])
            }
          }
        }
        n416 = Index Array(array=w807) -> (element=w804:i32)  [unwired: 1 in]
        n417 = Index Array(array=w819, index (row)=w804) -> (element=w818:dbl[])  [unwired: 1 in]
        n418 = Reverse 1D Array(array=w818) -> (reversed array=w817:dbl[])
        n419 = Index Array(array=w824, index=w804) -> (element=w823:cluster{"Ref X":refnum<vi>, "Ref Y":refnum<vi>})
        n420 = Index Array(array=w817) -> (element=w815:dbl)  [unwired: 1 in]
        n421 = Index Array(array=w806, index=w804) -> (element=w822:T1)
        n422 = Unbundle By Name(w823) -> ("Ref Y"=w811:refnum<vi>, "Ref X"=w810:refnum<vi>)
        n423 = Unbundle By Name(w822) -> ("Invert Direction Y"=w812:bool, "Invert Axis"=w816:bool, "Stepsize"=w813:dbl, "enable feedback"=w809:bool)
        n424 = Greater Or Equal To 0?(x=w815) -> (x >= 0?=w814:bool)
        n425 = call <vilib>:"Add State(s) to Queue__jki_lib_state_machine.vi"("State(s) in Front (\"\")"="Wait" ("State(s) in Front (\"\")"), "State(s) in (\"\")"=w828) -> ("States Out"=w827:string)  [unwired: 13 in]
        n426 = case shown="True" w809 {
          tunnel: w816 -> [_ w844]
          tunnel: w814 -> [_ w843]
          tunnel: w813 -> [_ w842]
          tunnel: w812 -> [_ w841]
          tunnel: w811 -> [_ w840]
          tunnel: w810 -> [_ w839]
          frame False {
          }
          frame True {
            n427 = case shown="True" w843 {
              tunnel: w841 -> [w852 w874]
              tunnel: w842 -> [w850 w872]
              tunnel: w844 -> [w849 w871]
              tunnel: w844 -> [w848 w870]
              tunnel: w840 -> [w846 w868]
              tunnel: w839 -> [w845 w867]
              frame True {
                n428 = case shown="False" w849 {
                  tunnel: [w863 w865] -> w851
                  tunnel: w846 -> [w864 _]
                  tunnel: w845 -> [_ w866]
                  frame False {
                    n429 = property class="DigNum (strict)"(reference=w864) -> ("Value"=w863:dbl)  [unwired: 1 in, 2 out]
                  }
                  frame True {
                    n430 = property class="DigNum (strict)"(reference=w866) -> ("Value"=w865:dbl)  [unwired: 1 in, 2 out]
                  }
                }
                n431 = case shown="False" w852 {
                  tunnel: w851 -> [w859 w862]
                  tunnel: w850 -> [w858 w861]
                  tunnel: [w857 w860] -> w847
                  frame False {
                    n432 = Add(x=w859, y=w858) -> (x+y=w857:dbl)
                  }
                  frame True {
                    n433 = Subtract(x=w862, y=w861) -> (x-y=w860:dbl)
                  }
                }
                n434 = case shown="False" w848 {
                  tunnel: w847 -> [w853 w855]
                  tunnel: w846 -> [w854 _]
                  tunnel: w845 -> [_ w856]
                  frame False {
                    n435 = property class="DigNum (strict)"(reference=w854, "Val(Sgnl)"=w853) -> ()  [unwired: 1 in, 2 out]
                  }
                  frame True {
                    n436 = property class="DigNum (strict)"(reference=w856, "Val(Sgnl)"=w855) -> ()  [unwired: 1 in, 2 out]
                  }
                }
              }
              frame False {
                n437 = case shown="False" w871 {
                  tunnel: [w885 w887] -> w873
                  tunnel: w868 -> [w886 _]
                  tunnel: w867 -> [_ w888]
                  frame False {
                    n438 = property class="DigNum (strict)"(reference=w886) -> ("Value"=w885:dbl)  [unwired: 1 in, 2 out]
                  }
                  frame True {
                    n439 = property class="DigNum (strict)"(reference=w888) -> ("Value"=w887:dbl)  [unwired: 1 in, 2 out]
                  }
                }
                n440 = case shown="False" w874 {
                  tunnel: w873 -> [w881 w884]
                  tunnel: w872 -> [w880 w883]
                  tunnel: [w879 w882] -> w869
                  frame False {
                    n441 = Subtract(x=w881, y=w880) -> (x-y=w879:dbl)
                  }
                  frame True {
                    n442 = Add(x=w884, y=w883) -> (x+y=w882:dbl)
                  }
                }
                n443 = case shown="False" w870 {
                  tunnel: w869 -> [w875 w877]
                  tunnel: w868 -> [w876 _]
                  tunnel: w867 -> [_ w878]
                  frame False {
                    n444 = property class="DigNum (strict)"(reference=w876, "Val(Sgnl)"=w875) -> ()  [unwired: 1 in, 2 out]
                  }
                  frame True {
                    n445 = property class="DigNum (strict)"(reference=w878, "Val(Sgnl)"=w877) -> ()  [unwired: 1 in, 2 out]
                  }
                }
              }
            }
          }
        }
        "Arguments Y" <- w821
      }
      frame "New Category: 2" {
        # "Your code here.\n(You can make a copy of, or modify, this frame)"
        n446 = call <vilib>:"Add State(s) to Queue__jki_lib_state_machine.vi"("State(s) in (\"\")"=w892) -> ("States Out"=w891:string)  [unwired: 14 in]
      }
      frame "Reset History" {
        # "Your code here.\n(You can make a copy of, or modify, this frame)"
        n447 = local read "Offset X"() -> (w895:dbl[][])
        n448 = Bundle By Name(cluster=w894, "Offset X"=w895, "Offset Y"=w895) -> (w893:T30)
        n449 = call <vilib>:"Add State(s) to Queue__jki_lib_state_machine.vi"("State(s) in (\"\")"=w898) -> ("States Out"=w897:string)  [unwired: 14 in]
      }
      frame "Save Config" {
        # "Your code here.\n(You can make a copy of, or modify, this frame)"
        n450 = Unbundle By Name(w914) -> ("move properties"=w900:T1[], "detection para"=w909:T6[])
        n451 = property on="motor config" class="Clust (strict)"() -> ("Value"=w908:T3)  [unwired: 2 in, 2 out]
        n452 = property on="Save Config" class="Bool (strict)"("Value"=FALSE ("Save Config")) -> ()  [unwired: 2 in, 2 out]
        n453 = call "File Dialog"("pattern (all files)"="*.cfg", "pattern label"="config") -> ("selected path"=w902:path)  [unwired: 10 in, 3 out]
        n454 = Bundle("move properties"=w900, "detection para"=w909, "Value"=w908) -> (w901:T8)  [unwired: 1 in]
        n455 = Open/Create/Replace File(file path (use dialog)=w902, error in=w906, operation (0:open)=T27."replace or create with confirmation") -> (refnum out=w910:refnum<file>, error out=w911:errorcluster)  [unwired: 3 in, 1 out]
        n456 = Write to Binary File(file (use dialog)=w910, data=w901, error in=w911) -> (refnum out=w913:refnum<file>, error out=w912:errorcluster)  [unwired: 3 in, 1 out]
        n457 = Close File(refnum=w913, error in=w912) -> (error out=w905:errorcluster)  [unwired: 1 out]
        n458 = call <vilib>:"Add State(s) to Queue__jki_lib_state_machine.vi"("State(s) in (\"\")"=w916) -> ("States Out"=w915:string)  [unwired: 14 in]
      }
      frame "Load Config" {
        # "Your code here.\n(You can make a copy of, or modify, this frame)"
        n459 = property on="Load Config" class="Bool (strict)"("Value"=FALSE ("Load Config")) -> ()  [unwired: 2 in, 2 out]
        n460 = call "File Dialog2"("pattern (all files)"="*.cfg", "pattern label"="config") -> ("selected path"=w925:path)  [unwired: 10 in, 3 out]
        n461 = Open/Create/Replace File(file path (use dialog)=w925, error in=w929, operation (0:open)=T27."open or create") -> (refnum out=w931:refnum<file>, error out=w932:errorcluster)  [unwired: 3 in, 1 out]
        n462 = Read from Binary File(5:"output cluster 2", 8:w932, 11:w931) -> (0:w933:errorcluster, 2:w924:T8, 3:w934:refnum<file>)  [unwired: 3 in, 1 out]
        n463 = Close File(refnum=w934, error in=w933) -> (error out=w928:errorcluster)  [unwired: 1 out]
        n464 = Unbundle By Name(w924) -> ("detection para"=w923:T6[], "move properties"=w920:T1[], "Value"=w921:T3)
        "move properties 3" <- w920
        n465 = call <vilib>:"Add State(s) to Queue__jki_lib_state_machine.vi"("State(s) in (\"\")"=w936) -> ("States Out"=w935:string)  [unwired: 14 in]
        n466 = property on="motor config" class="Clust (strict)"("Val(Sgnl)"=w921) -> ()  [unwired: 2 in, 2 out]
        n467 = Bundle By Name(cluster=w918, "detection para"=w923, "move properties"=w920) -> (w917:T30)
      }
      frame "Wait" {
        # "Your code here.\n(You can make a copy of, or modify, this frame)"
        n468 = Wait (ms)(milliseconds to wait=u32 300) -> ()  [unwired: 1 out]
        n469 = call <vilib>:"Add State(s) to Queue__jki_lib_state_machine.vi"("State(s) in (\"\")"=w943) -> ("States Out"=w942:string)  [unwired: 14 in]
        n470 = local read "Mean Centroid X"() -> (w938:dbl[][])
        n471 = Bundle By Name(cluster=w940, "Mean Centroid X"=w938, "Mean Centroid Y"=w938) -> (w939:T30)
      }
      frame "active" {
        # "Your code here.\n(You can make a copy of, or modify, this frame)"
        n472 = call-poly <userlib>:"Filter 1D Array__ogtk.vi"("items to filter"=w953, "array"=w949) -> ("filtered item indices"=w952:i32[])  [unwired: 4 in, 1 out]
        n473 = Unbundle By Name(w948) -> ("move properties"=w951:T1[], "detection para"=w946:T6[])  [unwired: 1 out]
        n474 = Index Array(array=w952) -> (element=w944:i32)  [unwired: 1 in]
        n475 = Index Array(array=w951, index=w944) -> (element=w950:T1)
        n476 = Index Array(array=w946, index=w944) -> (element=w945:T6)
        n477 = property on="move config" class="Clust (strict)"("Value"=w950) -> ()  [unwired: 2 in, 2 out]
        n478 = property on="beam detection para" class="Clust (strict)"("Value"=w945) -> ()  [unwired: 2 in, 2 out]
        n479 = Bundle By Name(cluster=w948, "active ccd"=w944) -> (w947:T30)
        n480 = call <vilib>:"Add State(s) to Queue__jki_lib_state_machine.vi"("State(s) in (\"\")"=w956) -> ("States Out"=w955:string)  [unwired: 14 in]
      }
      frame "Move Config" {
        # "Your code here.\n(You can make a copy of, or modify, this frame)"
        n481 = Unbundle By Name(w958) -> ("move properties"=w962:T1[], "active ccd"=w961:i32)
        n482 = Replace Array Subset(array=w962, new element="move config", index=w961) -> (w959:T1[])
        n483 = Bundle By Name(cluster=w958, "move properties"=w959) -> (w957:T30)
        n484 = call <vilib>:"Add State(s) to Queue__jki_lib_state_machine.vi"("State(s) in (\"\")"=w965) -> ("States Out"=w964:string)  [unwired: 14 in]
      }
      frame "Detection Config" {
        # "Your code here.\n(You can make a copy of, or modify, this frame)"
        n485 = Unbundle By Name(w970) -> ("detection para"=w966:T6[], "active ccd"=w971:i32)
        n486 = Replace Array Subset(array=w966, new element="beam detection para", index=w971) -> (w967:T6[])
        n487 = Bundle By Name(cluster=w970, "detection para"=w967) -> (w969:T30)
        n488 = call <vilib>:"Add State(s) to Queue__jki_lib_state_machine.vi"("State(s) in (\"\")"=w974) -> ("States Out"=w973:string)  [unwired: 14 in]
      }
      frame "Motor Config" {
        # "Your code here.\n(You can make a copy of, or modify, this frame)"
        n489 = Unbundle By Name("motor config") -> ("Motor CCD 1"=w991:u16, "Motor CCD 2"=w992:u16, "Motor CCD 3"=w993:u16, "Motor CCD 4"=w985:u16, "Motor CCD 5"=w984:u16, "Motor CCD 6"=w983:u16, "Motor CCD 7"=w982:u16, "Motor CCD 8"=w981:u16, "Motor CCD 9"=w980:u16, "Motor CCD 10"=w979:u16, "Motor CCD 11"=w978:u16, "Motor CCD 12"=w977:u16)
        n490 = local read "motor refs"() -> (w989:refnum<vi>[])
        n491 = Build Array(w991, w992, w993, w985, w984, w983, w982, w981, w980, w979, w978, w977) -> (w976:u16[])
        n492 = Increment(x=w976) -> (x+1=w975:u16[])
        n493 = for {
          tunnel: w975 -> [w1008] mode=indexing
          tunnel: w989 -> [w1003]
          tunnel: [w997] -> w988 mode=indexing
          n494 = Multiply(x=w1008, y=u16 3) -> (x*y=w1004:u16)
          n495 = Subtract(x=w1004, y=u16 3) -> (x-y=w1002:u16)
          n496 = Subtract(x=w1004, y=u16 2) -> (x-y=w1001:u16)
          n497 = Index Array(array=w1003, index=w1002) -> (element=w1000:refnum<vi>)
          n498 = Index Array(array=w1003, index=w1001) -> (element=w999:refnum<vi>)
          n499 = Bundle By Name(cluster="active Axis ref", "Ref X"=w1000, "Ref Y"=w999) -> (w997:cluster{"Ref X":refnum<vi>, "Ref Y":refnum<vi>})
        }
        n500 = call <vilib>:"Add State(s) to Queue__jki_lib_state_machine.vi"("State(s) in (\"\")"=w996) -> ("States Out"=w995:string)  [unwired: 14 in]
        n501 = Bundle By Name(cluster=w987, "active axis refs 2"=w988) -> (w986:T30)
      }
    }
    n502 = property on="Box" class="Arr (strict)"() -> ("Value"=w166:T2)  [unwired: 2 in, 2 out]
    n503 = for {
      tunnel: w169 -> [w190]
      tunnel: w168 -> [w191]
      tunnel: w167 -> [w183] mode=indexing
      tunnel: w166 -> [w184] mode=indexing
      n504 = call-poly <userlib>:"Filter 1D Array__ogtk.vi"("items to filter"=w183, "array"=w191) -> ("filtered item indices"=w192:i32[])  [unwired: 4 in, 1 out]
      n505 = Index Array(array=w192) -> (element=w186:i32)  [unwired: 1 in]
      n506 = Index Array(array=w190, index=w186) -> (element=w189:T22)
      n507 = Unbundle By Name(w189) -> ("Target.X::8"=w194:refnum<vi>, "Target.Y::8"=w193:refnum<vi>)
      n508 = property class="DigNum (strict)"(reference=w194) -> ("Value"=w188:dbl)  [unwired: 1 in, 2 out]
      n509 = property class="DigNum (strict)"(reference=w193) -> ("Value"=w187:dbl)  [unwired: 1 in, 2 out]
      n510 = call "draw crosshair imaq.vi"("Color"=u32 16774656, "Target.Y"=w187, "size"=35.0, "Target.X"=w188, "Bounding Rectangle"=T24 {"Left"=0, "Top"=0, "Right"=0, "Bottom"=0}, "image in"=w183) -> ("image out"=w182:T5)  [unwired: 5 in]
      n511 = call "draw box imaq.vi"("Color"=u32 1244928, "Rectangle"=w184, "image in"=w182) -> ()  [unwired: 8 in, 1 out]
    }
  }
  n512 = control-ref of="This Application"() -> (w148:refnum<vi>)
  n513 = control-ref of="This VI"() -> (w152:refnum<vi>)
  n514 = Current VI's Menubar() -> (w151:refnum<k9>)
  n515 = call "GUI_Master_subvi_reentrant_queues.vi"("This Application"=w148, "error in (no error)"=w149, "tcp data event"=w147, "Caller menu reference"=w151, "Caller VI ref"=w152) -> ("error out"=→"error IO 2":errorcluster)  [unwired: 6 in]
  n516 = for {
    tunnel: w58 -> [w1011] mode=indexing
    tunnel: w57 -> [w1010]
    tunnel: [w1009] -> w56 mode=indexing
    n517 = call "IMAQ Dispose"("Image"=w1011, "error in (no error)"=w1010) -> ("error out"=w1009:errorcluster)  [unwired: 4 in]
  }
  "Array" <- w56
